vi "secondary_user.vi"() -> ()   [LabVIEW 2014]
uses:
  <vilib>/addons/Modulation/Digital/General/MT Generate Bits (Galois, PN Order).vi
  <vilib>/Analysis/7linalg.llb/Complex Eigenvalues and Vectors.vi
  <vilib>/Analysis/2dsp.llb/Complex FFT.vi
  <vilib>/addons/Modulation/Analog/support/mod_Set Error Source.vi
  <vilib>/addons/Modulation/Digital/Support/Common/Validators/mod_Generate Bits Validate.vi
  var_stop.vi
  <vilib>/addons/Modulation/Digital/Support/Common/Validators/mod_Generate Filter Coefficients Validate.vi
  <vilib>/addons/Modulation/Digital/General/subVIs/mod_Generate Filter Coefficients.vi
  <vilib>/measure/maspectr.llb/FFT Power Spectrum and PSD for 1 Chan (CDB).vi
  <vilib>/addons/Modulation/Digital/General/MT Apply Matched Filter (Generic).vi
  <vilib>/addons/Modulation/Digital/General/MT Align to Ideal Symbols (Generic).vi
  <vilib>/Analysis/7linalg.llb/Create Special Real Matrix.vi
  <vilib>/Analysis/Matrix/Numeric/Multiply/Multiply - RM,R.vi
  <vilib>/Analysis/Matrix/Numeric/Conversions/Matrix To Array - RM.vi
  <instrlib>/niUSRP/niUSRP Fetch Rx Data (CDB Cluster).vi
  <vilib>/Analysis/2dsp.llb/AutoCorrelation Matrix (CDB).vi
  <vilib>/Analysis/Matrix/Numeric/Multiply/Multiply - CM,C.vi
  <vilib>/Analysis/Matrix/Numeric/Conversions/Matrix To Array - CM.vi
  <vilib>/measure/madcrms.llb/Averaged DC-RMS for 1 Chan.vi
  <instrlib>/niUSRP/niUSRP Write Tx Data (CDB Cluster).vi
  <vilib>/addons/Modulation/Digital/General/subVIs/mod_Generate Bits PN Sequence.vi
  <vilib>/addons/Modulation/Digital/General/MT Apply Pulse Shaping Filter (Generic).vi
  <vilib>/addons/Modulation/niDMT.lvlib
  <vilib>/measure/NI_MAPro.lvlib
  <vilib>/Analysis/Matrix/NI_Matrix.lvlib
  <vilib>/Analysis/NI_AALPro.lvlib
  <vilib>/Analysis/NI_AAL_SigProc.lvlib
panel:
  in  "packet bits 2":i32[](array[numeric])
  in  "random bits 2":i8[](array[numeric])
  in  "Gray code? 2":bool
  in  "Modulation 2":enum16{"PSK", "QAM"}(ring)=enum."QAM"
  in  "filter length (symbols) 2":i32=8 caption="filter length (symbols)"
  in  "filter parameter 2":dbl=0.5 caption="filter parameter" format="%.2f"
  in  "pulse shaping filter (none) 2":T1(ring)=enum."Raised Cosine" caption="pulse shaping filter (none)"
  in  "M-PSK (4) 2":i32=4 caption="M-ARY"
  in  "samples per symbol (16) 2":i32=4 caption="samples per symbol (16)"
  out "RX coerced gain 2":dbl format="%#_6f"
  out "RX coerced carrier frequency 2":dbl=915000000.0 format="%#_6p"
  out "RX coerced IQ rate  2":dbl=4000000.0 format="%#_6p"
  in  "RX active antenna 2":string="RX2"
  in  "RX gain 2":dbl format="%#_6f"
  in  "RX device names 2":refnum<k15>="192.168.10.2"
  out "TX coerced gain 2":dbl format="%#_6f"
  out "TX coerced carrier frequency 2":dbl=915000000.0 format="%#_6p"
  out "coerced IQ rate 2":dbl=4000000.0 format="%#_6p"
  in  "TX device names 2":refnum<k15>="192.168.10.2"
  in  "TX gain 2":dbl format="%#_6f"
  in  "carrier frequency 2":dbl=915000000.0 format="%#_6p"
  in  "IQ rate 2":dbl=400000.0 format="%#_6p"
  in  "stop 2":bool
  in  "Send (deprecated) 2":bool
  in  "random bits length 2":i32=50000
  out "Numeric 4":i32
  in  "millisecond multiple 2":u32=1000
  in  "Keep sending 2":bool=TRUE caption="Keep sending"
  out "packet bits length 2":i32
  in  "Transmit power (db) 2":dbl
  out "x = y? 2":bool
  out "Numeric 3":i32
  in  "number of samples 2":i64=40000
  out "# elements in queue 2":i32
  out "packet len 2":u32
  out "RX Constellation Map 2":cdb[](graph)
  out "RX Constellation Map (uneq) 2":cdb[](graph)
  out "valid? 2":bool
  out "Spectrum monitor 2":cluster{"f0":dbl, "df":dbl, "magnitude":dbl[]}(graph)={"f0"=-0.49993781867926873, "df"=0.00012436264146250465, "magnitude"=[]}
  out "found? 2":bool
  out "Rx String 2":string
  out "error bits 2":i32
  out "received bits 2":i32
  out "ber 2":dbl
  out "error symbols 2":i32
  out "received symbols 2":dbl
  out "ser 2":dbl
  in  "Ratio of  redundant 2":i32=5
  out "Detection Noise":dbl
  out "Primary User's average signal":dbl
  out "Delta of gain":dbl format="%#_6f"
  in  "Detection Mode":bool=TRUE
  out "Noise Average":dbl
  out "Signal Average":dbl
  in  "Average size":i32=10
  in  "Noise Threshold":dbl=-105.0 format="%#_6f"
  in  "matrix type(Dont Change), need to be indentity":i32
  in  "order of AC matrix":i32=8
  out "df":dbl
  out "f0":dbl
  out "my average power":dbl
  out "Average Noise floor in dBm per Hz":dbl
  out "Eigenvalues":cdb[](array[numeric]) format="%.2f"
  out "Min Eigenvalue method":bool
  out "Minimum eigenvalue method":dbl
  out "Energy of the Signal":dbl
  out "min eigen value":dbl
  out "max eigen value":dbl
  out "Waveform Graph 2":dbl[](graph)
  out "Waveform Graph":dbl[](graph)
  out "Power Spectrum / PSD":cluster{"f0":dbl, "df":dbl, "magnitude":dbl[]}(graph)
  out "data":waveform(cdb)
  out "Noise floor in dBm per Hz":dbl
  out "Energy of the Signal in dBm per Hz":dbl
  in  "Keep sending":bool=TRUE
  in  "millisecond multiple":u32=1000
  out "Numeric 2":i32
  out "Numeric":i32
  out "x = y?":bool
  in  "Ratio of  redundant":i32=5
  out "ser":dbl
  out "received symbols":dbl
  out "error symbols":i32
  in  "random bits length":i32=50000
  in  "packet bits":i32[](array[numeric])
  out "RX Constellation Map (uneq)":cdb[](graph)
  in  "Transmit power (db)":dbl
  out "ber":dbl
  out "received bits":i32
  out "error bits":i32
  in  "random bits":i8[](array[numeric])
  out "found?":bool
  out "# elements in queue":i32
  out "Spectrum monitor":cluster{"f0":dbl, "df":dbl, "magnitude":dbl[]}(graph)={"f0"=-0.49993781867926873, "df"=0.00012436264146250465, "magnitude"=[]}
  out "RX Constellation Map":cdb[](graph)
  out "valid?":bool
  in  "Gray code?":bool
  in  "Modulation":enum16{"PSK", "QAM"}(ring)=enum."QAM"
  out "Rx String":string
  out "packet len":u32
  in  "Send (deprecated)":bool
  in  "filter length (symbols)":i32=8
  in  "filter parameter":dbl=0.5 format="%.2f"
  in  "pulse shaping filter (none)":T1(ring)=enum."Raised Cosine"
  in  "M-PSK (4)":i32=4 caption="M-ARY"
  in  "samples per symbol (16)":i32=4
  out "packet bits length":i32
  in  "number of samples":i64=40000
  out "RX coerced gain":dbl format="%#_6f"
  out "RX coerced carrier frequency":dbl=915000000.0 format="%#_6p"
  out "RX coerced IQ rate":dbl=4000000.0 format="%#_6p"
  in  "RX active antenna":string="RX2"
  in  "RX gain":dbl format="%#_6f"
  in  "RX device names":refnum<k15>="192.168.10.3"
  out "TX coerced gain":dbl format="%#_6f"
  out "TX coerced carrier frequency":dbl=915000000.0 format="%#_6p"
  out "coerced IQ rate":dbl=4000000.0 format="%#_6p"
  in  "TX device names":refnum<k15>="192.168.10.3"
  in  "TX gain":dbl format="%#_6f"
  in  "carrier frequency":dbl=915000000.0 format="%#_6p"
  in  "IQ rate":dbl=800000.0 format="%#_6p"
  in  "stop":bool
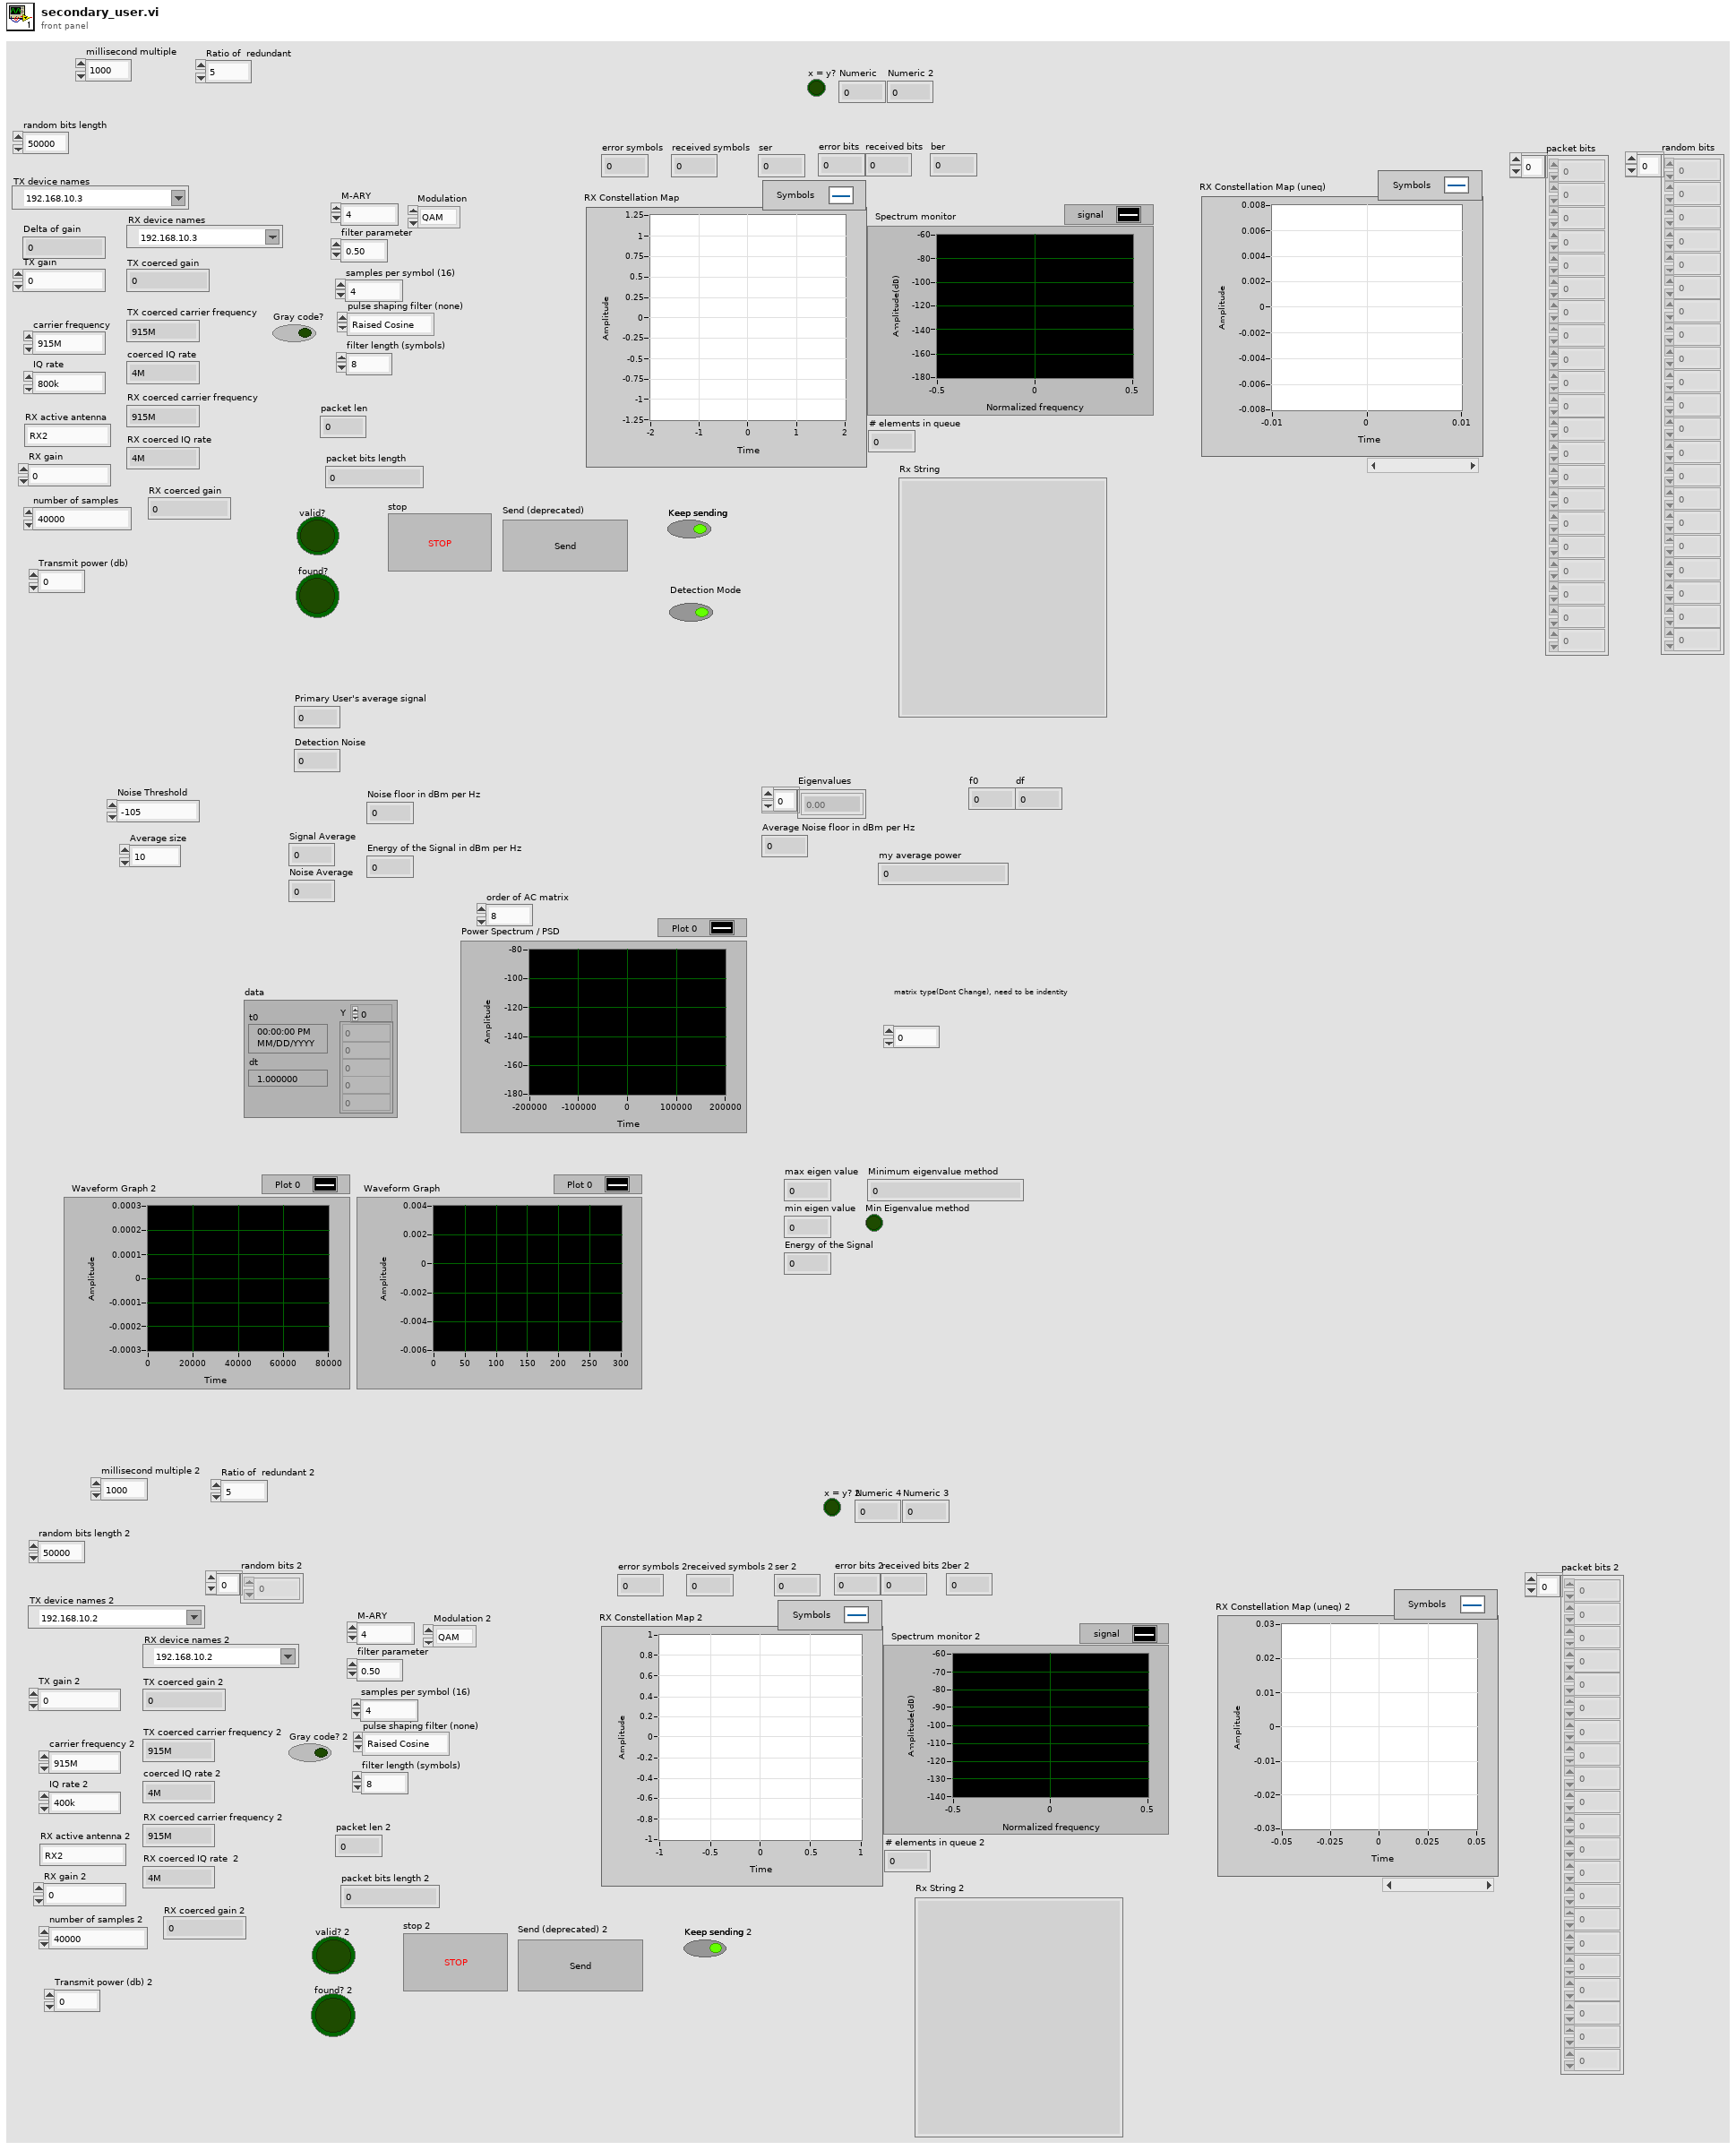
[diagram p1: front panel]
types:
  T1 = enum16{"none", "Raised Cosine", "Root Raised Cos", "Gaussian"}
  T2 = enum16{"FSK", "PSK", "QAM", "MSK", "PAM", "ASK", "CPM"}
  T3 = cluster{"samples per symbol (16)":i32, "symbol map":cdb[], "index map":u32[]}
  T4 = cluster{"samples per symbol (16)":i32, "symbol map":cdb[], i32[]}
  T5 = cluster{"samples per symbol (16) 2":i32, "symbol map":cdb[], "index map":u32[]}
  T6 = cluster{"samples per symbol (16) 2":i32, "symbol map":cdb[], i32[]}
  T7 = typedef "niAMT.lvlib/Complex Data Waveform.ctl" = cluster{"t0":dbl, "dt":dbl, "Y":cdb[]}
  T8 = typedef "NI_Matrix.lvlib/RealMatrix.ctl" = dbl[][]
  T9 = typedef "NI_Matrix.lvlib/ComplexMatrix.ctl" = cdb[][]
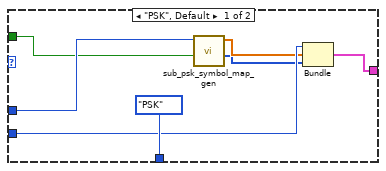
[diagram p2: hidden frame]
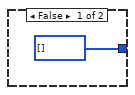
[diagram p5: hidden frame]
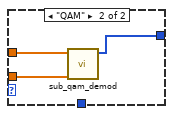
[diagram p6: hidden frame]
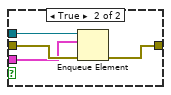
[diagram p10: hidden frame]
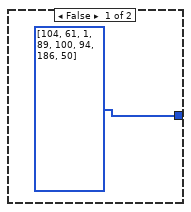
[diagram p13: hidden frame]
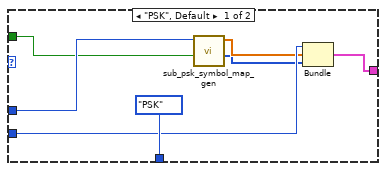
[diagram p18: hidden frame]
diagram:
  # "pre 64"
  # "Modulation"
  # "Filter"
  # "System Control"
  # "pre 64"
  # "Modulation"
  # "Filter"
  # "System Control"
  n1 = call <instrlib>:"niUSRP Open Rx Session.vi"("device names"="RX device names", "reset"=TRUE) -> ("session handle out"=w98:refnum<k15>, "error out"=w97:errorcluster)  [unwired: 12 in]
  n2 = call <instrlib>:"niUSRP Open Tx Session.vi"("device names"="TX device names", "reset"=TRUE) -> ("session handle out"=w110:refnum<k15>, "error out"=w109:errorcluster)  [unwired: 12 in]
  n3 = local read "Delta of gain"() -> (→"Delta of gain":dbl)
  n4 = call <instrlib>:"niUSRP Configure Signal.vi"("session handle"=w98, "IQ rate"="IQ rate", "carrier frequency"="carrier frequency", "gain"="RX gain", "error in (no error)"=w97, "active antenna"="RX active antenna") -> ("session handle out"=w89:refnum<k15>, "coerced IQ rate"=→"RX coerced IQ rate":dbl, "coerced carrier frequency"=→"RX coerced carrier frequency":dbl, "coerced gain"=→"RX coerced gain":dbl, "error out"=w73:errorcluster)  [unwired: 5 in]
  n5 = call <instrlib>:"niUSRP Open Rx Session.vi"("device names"="RX device names 2", "reset"=TRUE) -> ("session handle out"=w42:refnum<k15>, "error out"=w41:errorcluster)  [unwired: 12 in]
  n6 = call <instrlib>:"niUSRP Configure Signal.vi"("session handle"=w110, "IQ rate"="IQ rate", "carrier frequency"="carrier frequency", "gain"="TX gain", "error in (no error)"=w109, "active antenna"="TX1") -> ("session handle out"=w102:refnum<k15>, "coerced IQ rate"=w100:dbl, "coerced carrier frequency"=→"TX coerced carrier frequency":dbl, "coerced gain"=→"TX coerced gain":dbl, "error out"=w74:errorcluster)  [unwired: 5 in]
  "coerced IQ rate" <- w100
  n7 = case shown="\"QAM\"" "Modulation" {
    tunnel: [T2."PSK" ("modulation type") T2."QAM" ("modulation type")] -> w68
    tunnel: "M-PSK (4)" -> [w117 w123]
    tunnel: "Gray code?" -> [w116 w124]
    tunnel: "samples per symbol (16)" -> [w115 w122]
    tunnel: [w112 w119] -> w62
    frame "PSK", Default {
      n8 = call "sub_psk_symbol_map_gen.vi"("Gray code?"=w116, "M-PSK"=w117) -> ("index map"=w113:u32[], "symbol map"=w114:cdb[])  [unwired: 8 in]
      n9 = Bundle("samples per symbol (16)"=w115, "symbol map"=w114, "index map"=w113) -> (w112:T3)  [unwired: 1 in]
    }
    frame "QAM" {
      n10 = call "sub_qam_symbol_map_gen.vi"("Gray code?"=w124, "M-QAM"=w123) -> ("symbol map"=w121:cdb[])  [unwired: 9 in]
      n11 = Bundle("samples per symbol (16)"=w122, "symbol map"=w121, i32[] []) -> (w119:T4)  [unwired: 1 in]
    }
  }
  n12 = call <instrlib>:"niUSRP Open Tx Session.vi"("device names"="TX device names 2", "reset"=TRUE) -> ("session handle out"=w55:refnum<k15>, "error out"=w54:errorcluster)  [unwired: 12 in]
  n13 = call <vilib>:"MT Generate Filter Coefficients.vi"("pulse shaping filter (none)"="pulse shaping filter (none)", "modulation type"=w68, "pulse shaping samples per symbol (16)"="samples per symbol (16)", "matched samples per symbol (16)"="samples per symbol (16)", "filter parameter"="filter parameter", "filter length (symbols)"="filter length (symbols)") -> ("pulse shaping filter coefficients"=w79:dbl[], "matched filter coefficients"=w77:dbl[])  [unwired: 7 in, 1 out]
  n14 = call <instrlib>:"niUSRP Configure Signal.vi"("session handle"=w42, "IQ rate"="IQ rate 2", "carrier frequency"="carrier frequency 2", "gain"="RX gain 2", "error in (no error)"=w41, "active antenna"="RX active antenna 2") -> ("session handle out"=w33:refnum<k15>, "coerced IQ rate"=→"RX coerced IQ rate  2":dbl, "coerced carrier frequency"=→"RX coerced carrier frequency 2":dbl, "coerced gain"=→"RX coerced gain 2":dbl, "error out"=w17:errorcluster)  [unwired: 5 in]
  n15 = Unbundle(w62) -> ("symbol map"=w64:cdb[])  [unwired: 2 out]
  n16 = global write "var_stop.vi" "system stop"(FALSE) -> ()
  n17 = call "sub_bits_to_symbols.vi"("symbol map"=w64, "bits"=i16[] [1, 0, 1, 0, 1, 1, 0, 0, 1, 1, 0, 1, 1, 1, 0, 1, 1, 0, 1, 0, 0, 1, 0, 0, 1, 1, 1, 0, 0, 0, 1, 0, 1, 1, 1, 1, 0, 0, 1, 0, 1, 0, 0, 0, 1, 1, 0, 0, 0, 0, 1, 0, 0, 0, 0, 0, 1, 1, 1, 1, 1, 1, 0, 0] ("preamble(64) 2")) -> ("symbols"=w63:cdb[])  [unwired: 9 in]
  n18 = call <instrlib>:"niUSRP Configure Signal.vi"("session handle"=w55, "IQ rate"="IQ rate 2", "carrier frequency"="carrier frequency 2", "gain"="TX gain 2", "error in (no error)"=w54, "active antenna"="TX1") -> ("session handle out"=w46:refnum<k15>, "coerced IQ rate"=w44:dbl, "coerced carrier frequency"=→"TX coerced carrier frequency 2":dbl, "coerced gain"=→"TX coerced gain 2":dbl, "error out"=w18:errorcluster)  [unwired: 5 in]
  "coerced IQ rate 2" <- w44
  n19 = local write "packet bits"("packet bits") -> ()
  n20 = Divide(x="IQ rate", y="samples per symbol (16)") -> (x/y=w78:dbl)
  n21 = Merge Errors(w74, w73) -> (w72:errorcluster)
  n22 = local write "random bits"("random bits") -> ()
  n23 = case shown="\"QAM\"" "Modulation 2" {
    tunnel: [T2."PSK" ("modulation type") T2."QAM" ("modulation type")] -> w12
    tunnel: "M-PSK (4) 2" -> [w131 w137]
    tunnel: "Gray code? 2" -> [w130 w138]
    tunnel: "samples per symbol (16) 2" -> [w129 w136]
    tunnel: [w126 w133] -> w6
    frame "PSK", Default {
      n24 = call "sub_psk_symbol_map_gen.vi"("Gray code?"=w130, "M-PSK"=w131) -> ("index map"=w127:u32[], "symbol map"=w128:cdb[])  [unwired: 8 in]
      n25 = Bundle("samples per symbol (16) 2"=w129, "symbol map"=w128, "index map"=w127) -> (w126:T5)  [unwired: 1 in]
    }
    frame "QAM" {
      n26 = call "sub_qam_symbol_map_gen.vi"("Gray code?"=w138, "M-QAM"=w137) -> ("symbol map"=w135:cdb[])  [unwired: 9 in]
      n27 = Bundle("samples per symbol (16) 2"=w136, "symbol map"=w135, i32[] []) -> (w133:T6)  [unwired: 1 in]
    }
  }
  n28 = Reciprocal(x=w100) -> (1/x=w99:dbl)
  n29 = Obtain Queue(element data type=i8[] [] ("output bit stream")) -> (queue out=w84:refnum<queue>)  [unwired: 4 in, 2 out]
  n30 = Obtain Queue(element data type=i16[] []) -> (queue out=w111:refnum<queue>)  [unwired: 4 in, 2 out]
  n31 = Logarithm Base 2(1:"M-PSK (4)") -> (0:w59:dbl)
  n32 = Obtain Queue(element data type=cluster{"t0":dbl, "dt":dbl, "Y":cdb[]} {"t0"=0.0, "dt"=0.0, "Y"=[]} ("data")) -> (queue out=w88:refnum<queue>)  [unwired: 4 in, 2 out]
  n33 = Obtain Queue(element data type=cluster{"t0":dbl, "dt":dbl, "Y":cdb[]} {"t0"=0.0, "dt"=0.0, "Y"=[]} ("data")) -> (queue out=w85:refnum<queue>)  [unwired: 4 in, 2 out]
  n34 = Obtain Queue(element data type=cluster{"t0":dbl, "dt":dbl, "Y":cdb[]} {"t0"=0.0, "dt"=1.0, "Y"=[]} ("data")) -> (queue out=w103:refnum<queue>)  [unwired: 4 in, 2 out]
  n35 = call <vilib>:"MT Generate Filter Coefficients.vi"("pulse shaping filter (none)"="pulse shaping filter (none) 2", "modulation type"=w12, "pulse shaping samples per symbol (16)"="samples per symbol (16) 2", "matched samples per symbol (16)"="samples per symbol (16) 2", "filter parameter"="filter parameter 2", "filter length (symbols)"="filter length (symbols) 2") -> ("pulse shaping filter coefficients"=w23:dbl[], "matched filter coefficients"=w21:dbl[])  [unwired: 7 in, 1 out]
  n36 = case shown="No Error" w72 {
    tunnel: w111 -> [w190 _]
    tunnel: w103 -> [w185 _]
    tunnel: w102 -> [w186 _]
    tunnel: w99 -> [w144 _]
    tunnel: w89 -> [w175 _]
    tunnel: w88 -> [w169 _]
    tunnel: w85 -> [w165 _]
    tunnel: w84 -> [w163 _]
    tunnel: w62 -> [w157 _]
    tunnel: w79 -> [w160 _]
    tunnel: w78 -> [w159 _]
    tunnel: w77 -> [w158 _]
    tunnel: w63 -> [w151 _]
    tunnel: w59 -> [w149 _]
    frame No Error {
      w140 = 0
      w141 = 0.0
      w147 = 0
      w148 = 0
      # "USRP interface"
      n37 = call <instrlib>:"niUSRP Initiate.vi"("session handle"=w175, "error in (no error)"=errorcluster {"status"=FALSE, "code"=0, "source"=""}) -> ("session handle out"=w174:refnum<k15>, "error out"=w173:errorcluster)  [unwired: 12 in]
      n38 = while {
        tunnel: w163 -> [w212]
        shift-right: [w205] -> _
        shift-left: errorcluster {"status"=FALSE, "code"=0, "source"=""} ("error out") -> [w211]
        shift-right: [w200] -> _
        shift-left: w148 -> [w203]
        shift-right: [w201] -> _
        shift-left: w148 -> [w202]
        tunnel: w149 -> [w197]
        shift-right: [w194] -> _
        shift-left: w148 -> [w196]
        shift-right: [w193] -> _
        shift-left: w148 -> [w195]
        stop <- w210 stop-if-true
        n39 = Get Queue Status(queue=w212, error in (no error)=w211) -> (queue out=w207:refnum<queue>, error out=w206:errorcluster, # elements in queue=w209:i32)  [unwired: 1 in, 5 out]
        n40 = local read "packet bits length"() -> (w198:i32)
        n41 = local read "random bits"() -> (w204:i8[])
        n42 = Not Equal To 0?(x=w209) -> (x != 0?=w208:bool)
        n43 = case shown="True" w208 {
          tunnel: w207 -> [_ w254]
          tunnel: w206 -> [w217 w253]
          tunnel: [w217 w248] -> w205
          tunnel: w204 -> [_ w245]
          tunnel: w203 -> [w216 w241]
          tunnel: [w216 w240] -> w200
          tunnel: [w215 w238] -> w201
          tunnel: w202 -> [w215 w239]
          tunnel: w198 -> [_ w230]
          tunnel: w197 -> [_ w226]
          tunnel: w196 -> [w214 w222]
          tunnel: [w214 w221] -> w194
          tunnel: w195 -> [w213 w220]
          tunnel: [w213 w218] -> w193
          frame False {
          }
          frame True {
            w234 = 0
            w251 = 8 ("y")
            n44 = Dequeue Element(queue=w254, error in (no error)=w253) -> (element=w231:i8[], error out=w248:errorcluster)  [unwired: 1 in, 2 out]
            n45 = Array Size(array=w231) -> (size(s)=w225:i32)
            n46 = Subtract(x=w230, y=w225) -> (x-y=w229:i32)
            n47 = Array Subset(array=w245, index=0, length=w225) -> (w232:i8[])
            n48 = Quotient & Remainder(x=w229, y=w226) -> (x-y*floor(x/y)=w235:dbl)  [unwired: 1 out]
            n49 = Not Equal?(x=w232, y=w231) -> (x != y?=w244:bool[])
            n50 = Initialize Array(0, w235) -> (w233:i32[])
            n51 = Boolean To (0,1)(Boolean=w244) -> (0, 1=w243:i16[])
            n52 = Add Array Elements(numeric array=w243) -> (sum=w242:i16)
            n53 = Quotient & Remainder(x=w225, y=w226) -> (floor(x/y)=w219:dbl)  [unwired: 1 out]
            n54 = Insert Into Array(array=w233, index=w234, new element=w232) -> (w228:i32[])
            n55 = Insert Into Array(array=w233, index=w234, new element=w231) -> (w227:i32[])
            n56 = Quotient & Remainder(x=w225, y=w251) -> (floor(x/y)=w250:i32)  [unwired: 1 out]
            n57 = Add(x=w241, y=w242) -> (x+y=w240:i32)
            n58 = Add(x=w239, y=w225) -> (x+y=w238:i32)
            n59 = Not Equal To 0?(x=w231) -> (x != 0?=w252:bool[])
            n60 = Reshape Array(w228, w219, w226) -> (w224:i32[][])
            n61 = Reshape Array(w227, w219, w226) -> (w223:i32[][])
            n62 = Add(x=w219, y=w220) -> (x+y=w218:dbl)
            n63 = Reshape Array(w252, w250, w251) -> (w249:bool[][])
            n64 = for {
              tunnel: w224 -> [w262] mode=indexing
              tunnel: w223 -> [w263] mode=indexing
              shift-right: [w258] -> w221
              shift-left: w222 -> [w257]
              n65 = Not Equal?(x=w262, y=w263) -> (x != y?=w261:bool[])
              n66 = Boolean To (0,1)(Boolean=w261) -> (0, 1=w260:i16[])
              n67 = Add Array Elements(numeric array=w260) -> (sum=w259:i16)
              n68 = Not Equal To 0?(x=w259) -> (x != 0?=w256:bool)
              n69 = Boolean To (0,1)(Boolean=w256) -> (0, 1=w255:i16)
              n70 = Add(x=w255, y=w257) -> (x+y=w258:i32)
            }
            n71 = for {
              tunnel: w249 -> [w266] mode=indexing
              tunnel: [w265] -> w247 mode=indexing
              n72 = Boolean Array To Number(Boolean array=w266) -> (number=w264:u32)
              n73 = To Unsigned Byte Integer(number=w264) -> (unsigned 8bit integer=w265:u8)
            }
            n74 = Byte Array To String(unsigned byte array=w247) -> (string=→"Rx String":string)
          }
        }
        "error bits" <- w200
        "received bits" <- w201
        "error symbols" <- w194
        "received symbols" <- w193
        n75 = Divide(x=w194, y=w193) -> (x/y=→"ser":dbl)
        n76 = Divide(x=w200, y=w201) -> (x/y=→"ber":dbl)
        n77 = global read "var_stop.vi" "system stop"() -> (w210:bool)
      }
      n78 = while {
        tunnel: w169 -> [w359]
        shift-right: [w352] -> _
        shift-left: errorcluster {"status"=FALSE, "code"=0, "source"=""} ("error out") -> [w358]
        shift-right: [w338] -> _
        shift-left: cluster{"t0":dbl, "dt":dbl, "Y":cdb[]} {"t0"=0.0, "dt"=0.0, "Y"=[]} ("data") -> [w353]
        tunnel: w165 -> [w351]
        shift-right: [w350] -> _
        shift-left: errorcluster {"status"=FALSE, "code"=0, "source"=""} ("error out") -> [w349]
        stop <- w348 stop-if-true
        # "Energy\ndetector"
        n79 = Get Queue Status(queue=w359, error in (no error)=w358) -> (queue out=w354:refnum<queue>, error out=w355:errorcluster, # elements in queue=w357:i32)  [unwired: 1 in, 5 out]
        n80 = Not Equal To 0?(x=w357) -> (x != 0?=w356:bool)
        n81 = case shown="True" w356 {
          tunnel: w355 -> [w381 w392]
          tunnel: w354 -> [_ w391]
          tunnel: w353 -> [w380 w386]
          tunnel: [w381 w383] -> w352
          tunnel: [w380 w382] -> w345
          frame False {
          }
          frame True {
            n82 = Unbundle(w386) -> ("Y"=w389:cdb[])  [unwired: 2 out]
            n83 = Dequeue Element(queue=w391, error in (no error)=w392) -> (element=w390:cluster{"t0":dbl, "dt":dbl, "Y":cdb[]}, error out=w383:errorcluster)  [unwired: 1 in, 2 out]
            n84 = Unbundle(w390) -> ("t0"=w385:dbl, "dt"=w384:dbl, "Y"=w388:cdb[])
            n85 = Build Array (concatenate)(w389, w388) -> (w387:cdb[])
            n86 = Bundle(cluster=w386, "t0"=w385, "dt"=w384, "Y"=w387) -> (w382:cluster{"t0":dbl, "dt":dbl, "Y":cdb[]})
          }
        }
        n87 = call "rx_ed.vi"("Wavefrom"=w345) -> ("first pulse"=w335:i32, "length"=w346:i32[], "start index"=w347:i32[])  [unwired: 8 in]
        n88 = for {
          tunnel: w351 -> [w367]
          tunnel: w345 -> [w364]
          shift-right: [w366] -> w350
          shift-left: w349 -> [w365]
          tunnel: w347 -> [w363] mode=indexing
          tunnel: w346 -> [w362] mode=indexing
          tunnel: [w363] -> w341
          tunnel: [w362] -> w340
          n89 = Greater Or Equal?(x=w362, y=128) -> (x >= y?=w360:bool)
          n90 = case shown="True" w360 {
            tunnel: w367 -> [_ w379]
            tunnel: [w368 w378] -> w366
            tunnel: w365 -> [w368 w377]
            tunnel: w364 -> [_ w376]
            tunnel: w363 -> [_ w370]
            tunnel: w362 -> [_ w369]
            frame False {
            }
            frame True {
              n91 = Unbundle(w376) -> ("t0"=w374:dbl, "dt"=w375:dbl, "Y"=w372:cdb[])
              n92 = Array Subset(array=w372, index=w370, length=w369) -> (w371:cdb[])
              n93 = Bundle("t0"=w374, "dt"=w375, w371) -> (w373:cluster{"t0":dbl, "dt":dbl, cdb[]})  [unwired: 1 in]
              n94 = Enqueue Element(queue=w379, element=w373, error in (no error)=w377) -> (error out=w378:errorcluster)  [unwired: 1 in, 2 out]
            }
          }
        }
        n95 = Add(x=w341, y=w340) -> (x+y=w337:i32)
        n96 = Max & Min(x=w337, y=w335) -> (max(x,y)=w336:i32)  [unwired: 1 out]
        n97 = Unbundle(w345) -> ("t0"=w344:dbl, "dt"=w343:dbl, "Y"=w342:cdb[])
        n98 = global read "var_stop.vi" "system stop"() -> (w348:bool)
        n99 = Array Subset(array=w342, index=w336) -> (w339:cdb[])  [unwired: 1 in]
        n100 = Bundle(cluster=w345, "t0"=w344, "dt"=w343, "Y"=w339) -> (w338:cluster{"t0":dbl, "dt":dbl, "Y":cdb[]})
      }
      n101 = while {
        tunnel: w165 -> [w280]
        shift-right: [w274] -> _
        shift-left: errorcluster {"status"=FALSE, "code"=0, "source"=""} ("error out") -> [w279]
        tunnel: w163 -> [w273]
        shift-right: [w272] -> _
        shift-left: errorcluster {"status"=FALSE, "code"=0, "source"=""} ("error out") -> [w271]
        tunnel: w158 -> [w269]
        tunnel: w157 -> [w268]
        tunnel: w151 -> [w267]
        stop <- w270 stop-if-true
        # "Signal \nDemodulator"
        n102 = Get Queue Status(queue=w280, error in (no error)=w279) -> (queue out=w276:refnum<queue>, error out=w275:errorcluster, # elements in queue=w278:i32)  [unwired: 1 in, 5 out]
        n103 = Not Equal To 0?(x=w278) -> (x != 0?=w277:bool)
        n104 = case shown="True" w277 {
          tunnel: w276 -> [_ w313]
          tunnel: w275 -> [w282 w314]
          tunnel: [w282 w312] -> w274
          tunnel: w273 -> [_ w305]
          tunnel: [w281 w304] -> w272
          tunnel: w271 -> [w281 w303]
          tunnel: w269 -> [_ w292]
          tunnel: w268 -> [_ w296]
          tunnel: w267 -> [_ w288]
          frame False {
          }
          frame True {
            # "cross+eq"
            n105 = Unbundle(w296) -> ("samples per symbol (16)"=w295:i32, "symbol map"=w294:cdb[], "index map"=w293:u32[])
            n106 = Dequeue Element(queue=w313, error in (no error)=w314) -> (element=w287:cluster{"t0":dbl, "dt":dbl, "Y":cdb[]}, error out=w312:errorcluster)  [unwired: 1 in, 2 out]
            n107 = Unbundle(w287) -> ("Y"=w286:cdb[])  [unwired: 2 out]
            n108 = Bundle By Name("Y"=w286) -> (w291:waveform(cdb))  [unwired: 1 in]
            n109 = call-poly <vilib>:"FFT Power Spectrum and PSD.vi"("dB On (F)"=TRUE, "time signal"=w291) -> ("Power Spectrum / PSD"=→"Spectrum monitor":cluster{"f0":dbl, "df":dbl, "magnitude":dbl[]})  [unwired: 6 in, 3 out]
            n110 = call-poly <vilib>:"MT Matched Filter.vi"("input complex waveform"=w287, "matched filter coefficients"=w292, "samples per symbol (16)"=w295, "reset? (T)"=FALSE) -> ("output complex waveform"=w311:T7, "error out"=w310:errorcluster)  [unwired: 10 in]
            n111 = call-poly <vilib>:"MT Align To Ideal Symbols.vi"("input complex waveform"=w311, "matched filter coefficients"=w292, "samples per symbol (16)"=w295, "error in (no error)"=w310, "reset? (T)"=FALSE) -> ("output complex waveform"=w308:T7, "error out"=w309:errorcluster)  [unwired: 8 in, 1 out]
            n112 = call <vilib>:"MT Decimate Oversampled Waveform.vi"("input complex waveform"=w308, "decimation factor"=w295, "error in (no error)"=w309, "reset? (T)"=FALSE) -> ("output complex waveform"=w307:T7)  [unwired: 10 in, 1 out]
            n113 = Unbundle(w307) -> ("Y"=w285:cdb[])  [unwired: 2 out]
            n114 = call "rx_ceEq.vi"("preamble"=w288, "symbols"=w285) -> ("valid?"=w301:bool, "eq symbols"=w302:cdb[])
            "valid?" <- w301
            n115 = case shown="True" w301 {
              tunnel: [i8[] [] ("output bit stream") w319] -> w284
              tunnel: w294 -> [_ w320]
              tunnel: w302 -> [_ w317]
              tunnel: w293 -> [_ w318]
              tunnel: w285 -> [_ w316]
              frame False {
              }
              frame True {
                n116 = local read "Modulation"() -> (w321:enum16{"PSK", "QAM"})
                n117 = case shown="\"PSK\", Default" w321 {
                  tunnel: w317 -> [w325 w328]
                  tunnel: w320 -> [w324 w327]
                  tunnel: [w322 w326] -> w319
                  tunnel: w318 -> [w323 _]
                  frame "PSK", Default {
                    n118 = call "sub_psk_demod.vi"("index map"=w323, "symbol map"=w324, "symbol"=w325) -> ("bitstream"=w322:i16[])  [unwired: 8 in]
                  }
                  frame "QAM" {
                    n119 = call "sub_qam_demod.vi"("symbol map"=w327, "symbol"=w328) -> ("bitstream"=w326:i16[])  [unwired: 9 in]
                  }
                }
                "RX Constellation Map" <- w317
                "RX Constellation Map (uneq)" <- w316
              }
            }
            n120 = call "rx_pduExtract.vi"("output bit stream"=w284) -> ("found?"=w306:bool, "packet len"=w300:u32, "ppdu"=w283:i8[])  [unwired: 2 in]
            "found?" <- w306
            n121 = case shown="True" w306 {
              tunnel: w283 -> [_ w332]
              tunnel: w305 -> [_ w334]
              tunnel: [w329 w333] -> w304
              tunnel: w303 -> [w329 w330]
              tunnel: w300 -> [_ w331]
              frame False {
              }
              frame True {
                n122 = Enqueue Element(queue=w334, element=w332, error in (no error)=w330) -> (error out=w333:errorcluster)  [unwired: 1 in, 2 out]
                "packet len" <- w331
              }
            }
          }
        }
        n123 = global read "var_stop.vi" "system stop"() -> (w270:bool)
      }
      n124 = Initialize Array(cdb 0.0+0.0i, 25000 ("dimension size")) -> (w180:cdb[])
      n125 = Initialize Array(w141, w140) -> (w142:dbl[])
      n126 = while {
        tunnel: w190 -> [w690]
        shift-right: [w688] -> _
        shift-left: errorcluster {"status"=FALSE, "code"=0, "source"=""} ("error out") -> [w689]
        shift-right: [w686] -> _
        shift-left: -1111 -> [w687]
        shift-right: [w684] -> _
        shift-left: w147 -> [w685]
        tunnel: "Ratio of  redundant" -> [w683]
        stop <- "stop" stop-if-true
        n127 = local write "Detection Mode"("Detection Mode") -> ()
        n128 = Wait Until Next ms Multiple(millisecond multiple="millisecond multiple") -> ()  [unwired: 1 out]
        n129 = global write "var_stop.vi" "system stop"("stop") -> ()
        n130 = Not(x="Detection Mode") -> (.not. x?=w679:bool)
        n131 = And(x="Keep sending", y=w679) -> (x .and. y?=w681:bool)
        n132 = case shown="True" w681 {
          tunnel: w690 -> [_ w715]
          tunnel: w689 -> [w694 w714]
          tunnel: [w694 w713] -> w688
          tunnel: w687 -> [w693 w710]
          tunnel: [w693 w709] -> w686
          tunnel: w685 -> [w692 w695]
          tunnel: [w692 w700] -> w684
          tunnel: w683 -> [_ w701]
          frame False {
          }
          frame True {
            w707 = 8
            n133 = call-poly <vilib>:"MT Generate Bits (poly).vi"("total bits (128)"="random bits length", "seed in (0xD6BF7DF2)"=w710, "reset? (T)"=FALSE) -> ("output bit stream"=w697:i8[], "seed out"=w709:i32)  [unwired: 10 in, 1 out]
            n134 = Not Equal To 0?(x=w697) -> (x != 0?=w702:bool[])
            n135 = Array Size(array=w702) -> (size(s)=w706:i32)
            n136 = Divide(x=w706, y=w707) -> (x/y=w705:dbl)
            n137 = Reshape Array(w702, w705, w707) -> (w704:bool[][])
            n138 = for {
              tunnel: w704 -> [w720] mode=indexing
              tunnel: [w718] -> w703 mode=indexing
              n139 = Boolean Array To Number(Boolean array=w720) -> (number=w719:u32)
              n140 = To Unsigned Byte Integer(number=w719) -> (unsigned 8bit integer=w718:u8)
            }
            n141 = Increment(x=w695) -> (x+1=w700:i32)
            n142 = Array Size(array=w703) -> (size(s)=w712:i32)
            n143 = Quotient & Remainder(x=w695, y=w701) -> (x-y*floor(x/y)=w696:i32)  [unwired: 1 out]
            n144 = Not Equal To 0?(x=w712) -> (x != 0?=w716:bool)
            n145 = Equal?(x=w696, y=0) -> (x = y?=w698:bool)
            n146 = case shown="True" w716 {
              tunnel: w703 -> [_ w722]
              tunnel: w715 -> [_ w725]
              tunnel: w714 -> [w721 w724]
              tunnel: [w721 w723] -> w713
              frame False {
              }
              frame True {
                n147 = Enqueue Element(queue=w725, element=w722, error in (no error)=w724) -> (error out=w723:errorcluster)  [unwired: 1 in, 2 out]
              }
            }
            n148 = case shown="True" w698 {
              tunnel: w697 -> [_ w717]
              frame False {
              }
              frame True {
                n149 = local write "random bits"(w717) -> ()
              }
            }
            "Numeric" <- w695
          }
        }
      }
      n150 = while {
        tunnel: w174 -> [w513]
        shift-right: [w503] -> w170
        shift-left: w173 -> [w512]
        tunnel: w169 -> [w511]
        shift-right: [w505] -> _
        shift-left: errorcluster {"status"=FALSE, "code"=0, "source"=""} ("error out") -> [w510]
        tunnel: [w504] -> w171
        shift-right: [w447] -> _
        shift-left: errorcluster {"status"=FALSE, "code"=0, "source"=""} ("error out") -> [w448]
        shift-right: [w441] -> _
        shift-left: w141 -> [w442]
        shift-right: [w439] -> _
        shift-left: w140 -> [w440]
        tunnel: w144 -> [w435]
        tunnel: "Noise Threshold" -> [w422]
        shift-right: [w416] -> _
        shift-left: w142 -> [w420]
        shift-right: [w415] -> _
        shift-left: w142 -> [w419]
        shift-right: [w414] -> _
        shift-left: w141 -> [w418]
        shift-right: [w413] -> _
        shift-left: w141 -> [w417]
        shift-right: [w409] -> _
        shift-left: w141 -> [w411]
        shift-right: [w410] -> _
        shift-left: w141 -> [w397]
        shift-right: [w403] -> _
        shift-left: w140 -> [w405]
        shift-right: [w395] -> _
        shift-left: w141 -> [w396]
        i -> [w501]
        stop <- w502 stop-if-true
        # "USRP\nReceiver"
        n151 = local read "Detection Mode"() -> (w394:bool)
        n152 = Increment(x=w440) -> (x+1=w439:i32)
        n153 = Get Queue Status(queue=w511, error in (no error)=w510) -> (queue out=w507:refnum<queue>, error out=w506:errorcluster, # elements in queue=w509:i32)  [unwired: 1 in, 5 out]
        "# elements in queue" <- w509
        n154 = Less?(x=w509, y=5000) -> (x < y?=w499:bool)
        n155 = Greater Or Equal?(x=w501, y=25) -> (x >= y?=w498:bool)
        n156 = call-poly <vilib>:"Create Special Matrix.vi"("matrix type"="matrix type(Dont Change), need to be indentity", "matrix size"="order of AC matrix") -> ("Special Matrix"=w443:T8)  [unwired: 3 in, 1 out]
        n157 = And(x=w499, y=w498) -> (x .and. y?=w497:bool)
        n158 = call-poly <instrlib>:"niUSRP Fetch Rx Data (poly).vi"("session handle"=w513, "number of samples"="number of samples", "error in (no error)"=w512) -> ("session handle out"=w504:refnum<k15>, "data"=w462:cluster{"t0":dbl, "dt":dbl, "Y":cdb[]}, "error out"=w503:errorcluster)  [unwired: 9 in, 1 out]
        n159 = case shown="False" w497 {
          tunnel: w507 -> [_ w588]
          tunnel: w506 -> [w584 w587]
          tunnel: [w584 w586] -> w505
          tunnel: w462 -> [_ w585]
          frame False {
          }
          frame True {
            n160 = Enqueue Element(queue=w588, element=w585, error in (no error)=w587) -> (error out=w586:errorcluster)  [unwired: 1 in, 2 out]
          }
        }
        n161 = Unbundle(w462) -> ("dt"=w479:dbl, "Y"=w393:cdb[])  [unwired: 1 out]
        n162 = call-poly <vilib>:"AutoCorrelation Matrix.vi"("order"="order of AC matrix", "X"=w393) -> ("AutoCorrelation Matrix"=w444:T9)  [unwired: 8 in, 1 out]
        n163 = Absolute Value(x=w393) -> (abs(x)=w438:dbl[])
        n164 = Square(x=w438) -> (x^2=w481:dbl[])
        n165 = Add Array Elements(numeric array=w481) -> (sum=w473:dbl)
        "Energy of the Signal" <- w473
        n166 = Bundle By Name("Y"=w393, "dt"=w479) -> (w476:waveform(cdb))  [unwired: 1 in]
        "data" <- w476
        "Waveform Graph 2" <- w476
        n167 = Multiply(x=w473, y=w435) -> (x*y=w495:dbl)
        n168 = call-poly <vilib>:"Multiply.vi"("Complex Scalar c"=w435, "Complex Matrix A"=w444) -> ("A * c"=w487:T9)
        n169 = call-poly <vilib>:"Multiply.vi"("Real Scalar c"=2.05717e-20, "Real Matrix A"=w443) -> ("A * c"=w488:T8)
        n170 = Divide(x=w495, y="number of samples") -> (x/y=w463:dbl)
        n171 = call-poly <vilib>:"Matrix To Array.vi"("Complex Matrix"=w487) -> ("Complex 2D Array"=w489:cdb[][])
        n172 = call-poly <vilib>:"Matrix To Array.vi"("Real Matrix"=w488) -> ("Real 2D Array"=w490:dbl[][])
        n173 = Multiply(x=w463, y=1000.0) -> (x*y=w423:dbl)
        n174 = call-poly <vilib>:"FFT Power Spectrum and PSD.vi"("error in (no error)"=w448, "dB On (F)"=TRUE ("reset? (T)"), "time signal"=w476) -> ("error out"=w470:errorcluster, "Power Spectrum / PSD"=w449:cluster{"f0":dbl, "df":dbl, "magnitude":dbl[]})  [unwired: 5 in, 2 out]
        "Power Spectrum / PSD" <- w449
        n175 = Logarithm Base 10(1:w423) -> (0:w483:dbl)
        n176 = Logarithm Base 10(1:w423) -> (0:w425:dbl)
        n177 = Add(x=w489, y=w490) -> (x+y=w491:cdb[][])
        n178 = Multiply(x=w483, y=10.0) -> (x*y=→"Energy of the Signal in dBm per Hz":dbl)
        n179 = Multiply(x=w425, y=10.0) -> (x*y=w424:dbl)
        n180 = call-poly <vilib>:"Eigenvalues and Vectors.vi"("Input Matrix"=w491) -> ("Eigenvalues"=w492:cdb[])  [unwired: 2 in, 2 out]
        "Eigenvalues" <- w492
        n181 = Unbundle(w449) -> ("f0"=→"f0":dbl, "df"=→"df":dbl, "magnitude"=w456:dbl[])
        n182 = Absolute Value(x=w492) -> (abs(x)=w496:dbl[])
        n183 = Greater?(x=w424, y=w422) -> (0:w421:bool)
        n184 = case shown="True" w421 {
          tunnel: w420 -> [w544 w570]
          tunnel: w419 -> [w546 w566]
          tunnel: "Average size" -> [w545 w572]
          tunnel: w423 -> [w539 w563]
          tunnel: [w544 w567] -> w416
          tunnel: [w543 w566] -> w415
          tunnel: w418 -> [w542 w562]
          tunnel: w417 -> [w540 w565]
          tunnel: [w541 w565] -> w413
          tunnel: [w542 w564] -> w414
          tunnel: w405 -> [w537 w559]
          tunnel: w394 -> [_ w560]
          tunnel: [w537 w558] -> w403
          frame False {
            n185 = Add(x=w539, y=w540) -> (x+y=w538:dbl)
            n186 = Array Size(array=w546) -> (size(s)=w547:i32)
            n187 = Greater Or Equal?(x=w547, y=w545) -> (x >= y?=w548:bool)
            n188 = case shown="True" w548 {
              tunnel: w546 -> [w552 w557]
              tunnel: [w552 w556] -> w549
              tunnel: w538 -> [w551 w555]
              tunnel: [w551 w553] -> w541
              frame False {
              }
              frame True {
                n189 = Delete From Array(array=w557) -> (deleted portion=w554:dbl, array with subset deleted=w556:dbl[])  [unwired: 2 in]
                n190 = Subtract(x=w555, y=w554) -> (x-y=w553:dbl)
              }
            }
            n191 = Insert Into Array(array=w549, index=0, new element=w539) -> (w543:dbl[])
          }
          frame True {
            n192 = Array Size(array=w570) -> (size(s)=w573:i32)
            n193 = Add(x=w563, y=w562) -> (x+y=w561:dbl)
            n194 = Greater Or Equal?(x=w573, y=w572) -> (x >= y?=w571:bool)
            n195 = case shown="True" w571 {
              tunnel: w570 -> [w578 w583]
              tunnel: [w578 w582] -> w569
              tunnel: w561 -> [w577 w581]
              tunnel: [w577 w579] -> w564
              frame False {
              }
              frame True {
                n196 = Delete From Array(array=w583) -> (deleted portion=w580:dbl, array with subset deleted=w582:dbl[])  [unwired: 2 in]
                n197 = Subtract(x=w581, y=w580) -> (x-y=w579:dbl)
              }
            }
            n198 = case shown="False" w560 {
              tunnel: [w574 w576] -> w558
              tunnel: w559 -> [w575 w576]
              frame False {
                n199 = Increment(x=w575) -> (x+1=w574:i32)
              }
              frame True {
              }
            }
            n200 = Insert Into Array(array=w569, index=0, new element=w563) -> (w567:dbl[])
          }
        }
        n201 = Divide(x=w456, y=10.0) -> (x/y=w457:dbl[])
        n202 = Array Max & Min(array=w496) -> (max value=→"max eigen value":dbl, min value=w468:dbl)  [unwired: 2 out]
        "min eigen value" <- w468
        n203 = call-poly <vilib>:"Averaged DC-RMS.vi"("error in (no error)"=w470, "signal in"=w476) -> ("error out"=w447:errorcluster)  [unwired: 5 in, 4 out]
        n204 = Array Size(array=w456) -> (size(s)=w460:i32)
        n205 = Divide(x=w473, y=w468) -> (x/y=w437:dbl)
        "Minimum eigenvalue method" <- w437
        n206 = Power Of 10(x=w457) -> (10^x=w454:dbl[])
        n207 = Logarithm Base 10(1:w468) -> (0:w493:dbl)
        n208 = Greater?(x=w437, y=800000000000000.0) -> (0:→"Min Eigenvalue method":bool)
        n209 = Add Array Elements(numeric array=w454) -> (sum=w461:dbl)
        n210 = call-poly <vilib>:"FFT.vi"("FFT size"=256, "shift?"=FALSE, "X"=w393) -> ("FFT {X}"=→"Waveform Graph":cdb[])  [unwired: 7 in, 1 out]
        n211 = Divide(x=w461, y=w460) -> (x/y=w453:dbl)
        n212 = Multiply(x=w493, y=10.0) -> (x*y=→"Noise floor in dBm per Hz":dbl)
        n213 = Logarithm Base 10(1:w453) -> (0:w452:dbl)
        n214 = Array Size(array=w416) -> (size(s)=w429:i32)
        n215 = Multiply(x=w452, y=10.0) -> (x*y=→"my average power":dbl)
        n216 = Quotient & Remainder(x=w403, y="Average size") -> (x-y*floor(x/y)=w402:i32)  [unwired: 1 out]
        n217 = Divide(x=w414, y=w429) -> (x/y=w430:dbl)
        n218 = Equal To 0?(x=w402) -> (x = 0?=w400:bool)
        n219 = Not Equal To 0?(x=w397) -> (x != 0?=w408:bool)
        n220 = Logarithm Base 10(1:w430) -> (0:w433:dbl)
        n221 = And(x=w394, y=w408) -> (x .and. y?=w406:bool)
        n222 = global read "var_stop.vi" "system stop"() -> (w502:bool)
        n223 = Multiply(x=w433, y=10.0) -> (x*y=w398:dbl)
        "Signal Average" <- w398
        n224 = Add(x=w468, y=w442) -> (x+y=w441:dbl)
        n225 = Not Equal To 0?(x=w398) -> (x != 0?=w407:bool)
        n226 = Divide(x=w441, y=w439) -> (x/y=w467:dbl)
        n227 = And(x=w407, y=w406) -> (x .and. y?=w401:bool)
        n228 = Logarithm Base 10(1:w467) -> (0:w466:dbl)
        n229 = Array Size(array=w415) -> (size(s)=w428:i32)
        n230 = And(x=w400, y=w401) -> (x .and. y?=w399:bool)
        n231 = Multiply(x=w466, y=10.0) -> (x*y=→"Average Noise floor in dBm per Hz":dbl)
        n232 = case shown="True" w399 {
          tunnel: w398 -> [_ w524]
          tunnel: w397 -> [_ w523]
          tunnel: w396 -> [w514 w520]
          tunnel: [w514 w515] -> w395
          frame False {
          }
          frame True {
            n233 = Subtract(x=w524, y=w523) -> (x-y=w517:dbl)
            n234 = Greater Than 0?(x=w517) -> (x > 0?=w522:bool)
            n235 = Add(x=w517, y=10.0) -> (x+y=w519:dbl)
            n236 = case shown="True" w522 {
              tunnel: w517 -> [_ w531]
              tunnel: w520 -> [w529 w532]
              tunnel: [w529 w530] -> w516
              frame False {
              }
              frame True {
                n237 = Subtract(x=w532, y=w531) -> (x-y=w530:dbl)
              }
            }
            n238 = Less Than 0?(x=w519) -> (x < 0?=w518:bool)
            n239 = case shown="False" w518 {
              tunnel: w517 -> [_ w527]
              tunnel: w516 -> [w525 w528]
              tunnel: [w525 w526] -> w515
              frame False {
              }
              frame True {
                n240 = Subtract(x=w528, y=w527) -> (x-y=w526:dbl)
              }
            }
          }
        }
        n241 = Divide(x=w413, y=w428) -> (x/y=w427:dbl)
        n242 = Logarithm Base 10(1:w427) -> (0:w431:dbl)
        n243 = Multiply(x=w431, y=10.0) -> (x*y=w412:dbl)
        "Noise Average" <- w412
        n244 = case shown="True" w394 {
          tunnel: w398 -> [_ w536]
          tunnel: w412 -> [_ w535]
          tunnel: w411 -> [w534 _]
          tunnel: [w533 w535] -> w410
          tunnel: w397 -> [w533 _]
          tunnel: [w534 w536] -> w409
          frame False {
          }
          frame True {
          }
        }
        "Primary User's average signal" <- w409
        "Detection Noise" <- w410
        n245 = local write "Delta of gain"(w395) -> ()
      }
      n246 = Bundle(0.0, w144, w180) -> (w178:cluster{dbl, dbl, cdb[]})  [unwired: 1 in]
      n247 = while {
        shift-right: [w598] -> w189
        shift-left: errorcluster {"status"=FALSE, "code"=0, "source"=""} ("error out") -> [w596]
        tunnel: [w597] -> w188
        tunnel: w186 -> [w595]
        tunnel: w185 -> [w593]
        shift-right: [w591] -> _
        shift-left: errorcluster {"status"=FALSE, "code"=0, "source"=""} ("error out") -> [w592]
        tunnel: w178 -> [w590]
        stop <- w589 stop-if-true
        # "USRP\nTransmitter"
        n248 = Get Queue Status(queue=w593, error in (no error)=w592) -> (queue out=w600:refnum<queue>, error out=w599:errorcluster, # elements in queue=w602:i32)  [unwired: 1 in, 5 out]
        n249 = Not Equal To 0?(x=w602) -> (x != 0?=w601:bool)
        n250 = case shown="True" w601 {
          tunnel: w600 -> [_ w608]
          tunnel: w599 -> [w603 w607]
          tunnel: [w604 w606] -> w594
          tunnel: [w603 w605] -> w591
          tunnel: w590 -> [w604 _]
          frame False {
          }
          frame True {
            n251 = Dequeue Element(queue=w608, error in (no error)=w607) -> (element=w606:cluster{"t0":dbl, "dt":dbl, "Y":cdb[]}, error out=w605:errorcluster)  [unwired: 1 in, 2 out]
          }
        }
        n252 = global read "var_stop.vi" "system stop"() -> (w589:bool)
        n253 = call-poly <instrlib>:"niUSRP Write Tx Data (poly).vi"("session handle"=w595, "data"=w594, "error in (no error)"=w596) -> ("session handle out"=w597:refnum<k15>, "error out"=w598:errorcluster)  [unwired: 11 in]
      }
      n254 = call <instrlib>:"niUSRP Close Session.vi"("session handle"=w188, "error in (no error)"=w189) -> ()  [unwired: 13 in, 1 out]
      n255 = Initialize Array(cdb 0.0+0.0i, 1024 ("dimension size")) -> (w152:cdb[])
      n256 = while {
        tunnel: w190 -> [w623]
        shift-right: [w620] -> _
        shift-left: errorcluster {"status"=FALSE, "code"=0, "source"=""} ("error out") -> [w626]
        tunnel: w185 -> [w619]
        shift-right: [w618] -> _
        shift-left: errorcluster {"status"=FALSE, "code"=0, "source"=""} ("error out") -> [w617]
        tunnel: w157 -> [w615]
        tunnel: w160 -> [w614]
        tunnel: w159 -> [w613]
        tunnel: w152 -> [w612]
        shift-right: [w610] -> _
        shift-left: w147 -> [w611]
        tunnel: "Ratio of  redundant" -> [w609]
        stop <- w616 stop-if-true
        n257 = Get Queue Status(queue=w623, error in (no error)=w626) -> (queue out=w621:refnum<queue>, error out=w622:errorcluster, # elements in queue=w625:i32)  [unwired: 1 in, 5 out]
        n258 = Not Equal To 0?(x=w625) -> (x != 0?=w624:bool)
        n259 = case shown="True" w624 {
          tunnel: w622 -> [w629 w672]
          tunnel: w621 -> [_ w671]
          tunnel: [w629 w670] -> w620
          tunnel: w619 -> [_ w665]
          tunnel: [w628 w664] -> w618
          tunnel: w617 -> [w628 w663]
          tunnel: w615 -> [_ w661]
          tunnel: w614 -> [_ w660]
          tunnel: w613 -> [_ w659]
          tunnel: w612 -> [_ w649]
          tunnel: w611 -> [w627 w634]
          tunnel: [w627 w636] -> w610
          tunnel: w609 -> [_ w631]
          frame False {
          }
          frame True {
            # "length"
            # "Waveform \nGenerator"
            n260 = Dequeue Element(queue=w671, error in (no error)=w672) -> (element=w646:i16[], error out=w670:errorcluster)  [unwired: 1 in, 2 out]
            n261 = Quotient & Remainder(x=w634, y=w631) -> (x-y*floor(x/y)=w630:i32)  [unwired: 1 out]
            n262 = Unbundle(w661) -> ("samples per symbol (16)"=w655:i32, "symbol map"=w648:cdb[])  [unwired: 1 out]
            n263 = Equal?(x=w630, y=0) -> (x = y?=w632:bool)
            "x = y?" <- w632
            n264 = case shown="True" w632 {
              tunnel: [u8[] [104, 61, 1, 89, 100, 94, 186, 50] ("Array 2") u8[] [53, 187, 37, 71, 79, 49, 4, 63] ("Array 2")] -> w635
              frame False {
              }
              frame True {
              }
            }
            n265 = Increment(x=w634) -> (x+1=w636:i32)
            n266 = Array Size(array=w646) -> (size(s)=w657:i32)
            n267 = To Unsigned Word Integer(number=w657) -> (unsigned 16bit integer=w656:u16)
            n268 = Number To Boolean Array(number=w656) -> (Boolean array=w669:bool[])
            n269 = Reshape Array(w669, 2 ("dimension size"), 8 ("dimension size")) -> (w666:bool[][])
            n270 = for {
              tunnel: w666 -> [w677] mode=indexing
              tunnel: [w675] -> w658 mode=indexing
              n271 = Boolean Array To Number(Boolean array=w677) -> (number=w676:u32)
              n272 = To Unsigned Byte Integer(number=w676) -> (unsigned 8bit integer=w675:u8)
            }
            n273 = Build Array (concatenate)(w635, w658, w658, w646) -> (w662:i16[])
            n274 = call "tx_pduGen.vi"("byte array"=w662) -> ("packet bits length"=w637:i32, "pdu"=w639:i32[])  [unwired: 3 in]
            "packet bits length" <- w637
            n275 = local write "packet bits"(w639) -> ()
            n276 = local write "packet bits length"(w637) -> ()
            n277 = call "sub_bits_to_symbols.vi"("symbol map"=w648, "bits"=w639) -> ("symbols"=w647:cdb[])  [unwired: 9 in]
            n278 = Build Array (concatenate)(w647, w649) -> (w645:cdb[])
            n279 = call-poly <vilib>:"MT Pulse Shaping Filter.vi"("symbols"=w645, "pulse shaping filter coefficients"=w660, "samples per symbol (16)"=w655, "symbol rate (Hz)"=w659, "reset? (T)"=FALSE) -> ("output complex waveform"=w654:T7)  [unwired: 9 in, 1 out]
            n280 = Divide(x="Transmit power (db)", y=20.0) -> (x/y=w642:dbl)
            n281 = Unbundle(w654) -> ("t0"=w653:dbl, "dt"=w652:dbl, "Y"=w641:cdb[])
            n282 = Power Of 10(x=w642) -> (10^x=w640:dbl)
            n283 = Multiply(x=w641, y=w640) -> (x*y=w638:cdb[])
            n284 = Bundle(cluster=w654, "t0"=w653, "dt"=w652, "Y"=w638) -> (w651:T7)
            n285 = Enqueue Element(queue=w665, element=w651, error in (no error)=w663) -> (error out=w664:errorcluster)  [unwired: 1 in, 2 out]
            "Numeric 2" <- w634
          }
        }
        n286 = global read "var_stop.vi" "system stop"() -> (w616:bool)
      }
      n287 = call <instrlib>:"niUSRP Abort.vi"("session handle"=w171, "error in (no error)"=w170) -> ("session handle out"=w177:refnum<k15>, "error out"=w176:errorcluster)  [unwired: 12 in]
      n288 = call <instrlib>:"niUSRP Close Session.vi"("session handle"=w177, "error in (no error)"=w176) -> ()  [unwired: 13 in, 1 out]
    }
    frame Error {
    }
  }
  n289 = Unbundle(w6) -> ("symbol map"=w8:cdb[])  [unwired: 2 out]
  n290 = global write "var_stop.vi" "system stop"(FALSE) -> ()
  n291 = call "sub_bits_to_symbols.vi"("symbol map"=w8, "bits"=i16[] [1, 0, 1, 0, 1, 1, 0, 0, 1, 1, 0, 1, 1, 1, 0, 1, 1, 0, 1, 0, 0, 1, 0, 0, 1, 1, 1, 0, 0, 0, 1, 0, 1, 1, 1, 1, 0, 0, 1, 0, 1, 0, 0, 0, 1, 1, 0, 0, 0, 0, 1, 0, 0, 0, 0, 0, 1, 1, 1, 1, 1, 1, 0, 0] ("preamble(64) 2")) -> ("symbols"=w7:cdb[])  [unwired: 9 in]
  n292 = local write "packet bits 2"("packet bits 2") -> ()
  n293 = local write "random bits 2"("random bits 2") -> ()
  n294 = Divide(x="IQ rate 2", y="samples per symbol (16) 2") -> (x/y=w22:dbl)
  n295 = Merge Errors(w18, w17) -> (w16:errorcluster)
  n296 = Reciprocal(x=w44) -> (1/x=w43:dbl)
  n297 = Obtain Queue(element data type=i8[] [] ("output bit stream")) -> (queue out=w28:refnum<queue>)  [unwired: 4 in, 2 out]
  n298 = Obtain Queue(element data type=i16[] []) -> (queue out=w56:refnum<queue>)  [unwired: 4 in, 2 out]
  n299 = Logarithm Base 2(1:"M-PSK (4) 2") -> (0:w3:dbl)
  n300 = Obtain Queue(element data type=cluster{"t0":dbl, "dt":dbl, "Y":cdb[]} {"t0"=0.0, "dt"=0.0, "Y"=[]} ("data")) -> (queue out=w32:refnum<queue>)  [unwired: 4 in, 2 out]
  n301 = Obtain Queue(element data type=cluster{"t0":dbl, "dt":dbl, "Y":cdb[]} {"t0"=0.0, "dt"=0.0, "Y"=[]} ("data")) -> (queue out=w29:refnum<queue>)  [unwired: 4 in, 2 out]
  n302 = Obtain Queue(element data type=cluster{"t0":dbl, "dt":dbl, "Y":cdb[]} {"t0"=0.0, "dt"=1.0, "Y"=[]} ("data")) -> (queue out=w47:refnum<queue>)  [unwired: 4 in, 2 out]
  n303 = case shown="No Error" w16 {
    tunnel: w56 -> [w771 _]
    tunnel: w47 -> [w766 _]
    tunnel: w46 -> [w767 _]
    tunnel: w43 -> [w760 _]
    tunnel: w33 -> [w755 _]
    tunnel: w32 -> [w749 _]
    tunnel: w29 -> [w745 _]
    tunnel: w28 -> [w743 _]
    tunnel: w6 -> [w737 _]
    tunnel: w23 -> [w740 _]
    tunnel: w22 -> [w739 _]
    tunnel: w21 -> [w738 _]
    tunnel: w7 -> [w731 _]
    tunnel: w3 -> [w729 _]
    frame No Error {
      w727 = 0
      w728 = 0
      # "USRP interface"
      n304 = call <instrlib>:"niUSRP Initiate.vi"("session handle"=w755, "error in (no error)"=errorcluster {"status"=FALSE, "code"=0, "source"=""}) -> ("session handle out"=w754:refnum<k15>, "error out"=w753:errorcluster)  [unwired: 12 in]
      n305 = while {
        tunnel: w743 -> [w793]
        shift-right: [w786] -> _
        shift-left: errorcluster {"status"=FALSE, "code"=0, "source"=""} ("error out") -> [w792]
        shift-right: [w781] -> _
        shift-left: w728 -> [w784]
        shift-right: [w782] -> _
        shift-left: w728 -> [w783]
        tunnel: w729 -> [w778]
        shift-right: [w775] -> _
        shift-left: w728 -> [w777]
        shift-right: [w774] -> _
        shift-left: w728 -> [w776]
        stop <- w791 stop-if-true
        n306 = Get Queue Status(queue=w793, error in (no error)=w792) -> (queue out=w788:refnum<queue>, error out=w787:errorcluster, # elements in queue=w790:i32)  [unwired: 1 in, 5 out]
        n307 = local read "packet bits length 2"() -> (w779:i32)
        n308 = local read "random bits 2"() -> (w785:i8[])
        n309 = Not Equal To 0?(x=w790) -> (x != 0?=w789:bool)
        n310 = case shown="True" w789 {
          tunnel: w788 -> [_ w835]
          tunnel: w787 -> [w798 w834]
          tunnel: [w798 w829] -> w786
          tunnel: w785 -> [_ w826]
          tunnel: w784 -> [w797 w822]
          tunnel: [w797 w821] -> w781
          tunnel: [w796 w819] -> w782
          tunnel: w783 -> [w796 w820]
          tunnel: w779 -> [_ w811]
          tunnel: w778 -> [_ w807]
          tunnel: w777 -> [w795 w803]
          tunnel: [w795 w802] -> w775
          tunnel: w776 -> [w794 w801]
          tunnel: [w794 w799] -> w774
          frame False {
          }
          frame True {
            w815 = 0
            w832 = 8 ("y")
            n311 = Dequeue Element(queue=w835, error in (no error)=w834) -> (element=w812:i8[], error out=w829:errorcluster)  [unwired: 1 in, 2 out]
            n312 = Array Size(array=w812) -> (size(s)=w806:i32)
            n313 = Subtract(x=w811, y=w806) -> (x-y=w810:i32)
            n314 = Array Subset(array=w826, index=0, length=w806) -> (w813:i8[])
            n315 = Quotient & Remainder(x=w810, y=w807) -> (x-y*floor(x/y)=w816:dbl)  [unwired: 1 out]
            n316 = Not Equal?(x=w813, y=w812) -> (x != y?=w825:bool[])
            n317 = Initialize Array(0, w816) -> (w814:i32[])
            n318 = Boolean To (0,1)(Boolean=w825) -> (0, 1=w824:i16[])
            n319 = Add Array Elements(numeric array=w824) -> (sum=w823:i16)
            n320 = Quotient & Remainder(x=w806, y=w807) -> (floor(x/y)=w800:dbl)  [unwired: 1 out]
            n321 = Insert Into Array(array=w814, index=w815, new element=w813) -> (w809:i32[])
            n322 = Insert Into Array(array=w814, index=w815, new element=w812) -> (w808:i32[])
            n323 = Quotient & Remainder(x=w806, y=w832) -> (floor(x/y)=w831:i32)  [unwired: 1 out]
            n324 = Add(x=w822, y=w823) -> (x+y=w821:i32)
            n325 = Add(x=w820, y=w806) -> (x+y=w819:i32)
            n326 = Not Equal To 0?(x=w812) -> (x != 0?=w833:bool[])
            n327 = Reshape Array(w809, w800, w807) -> (w805:i32[][])
            n328 = Reshape Array(w808, w800, w807) -> (w804:i32[][])
            n329 = Add(x=w800, y=w801) -> (x+y=w799:dbl)
            n330 = Reshape Array(w833, w831, w832) -> (w830:bool[][])
            n331 = for {
              tunnel: w805 -> [w843] mode=indexing
              tunnel: w804 -> [w844] mode=indexing
              shift-right: [w839] -> w802
              shift-left: w803 -> [w838]
              n332 = Not Equal?(x=w843, y=w844) -> (x != y?=w842:bool[])
              n333 = Boolean To (0,1)(Boolean=w842) -> (0, 1=w841:i16[])
              n334 = Add Array Elements(numeric array=w841) -> (sum=w840:i16)
              n335 = Not Equal To 0?(x=w840) -> (x != 0?=w837:bool)
              n336 = Boolean To (0,1)(Boolean=w837) -> (0, 1=w836:i16)
              n337 = Add(x=w836, y=w838) -> (x+y=w839:i32)
            }
            n338 = for {
              tunnel: w830 -> [w847] mode=indexing
              tunnel: [w846] -> w828 mode=indexing
              n339 = Boolean Array To Number(Boolean array=w847) -> (number=w845:u32)
              n340 = To Unsigned Byte Integer(number=w845) -> (unsigned 8bit integer=w846:u8)
            }
            n341 = Byte Array To String(unsigned byte array=w828) -> (string=→"Rx String 2":string)
          }
        }
        "error bits 2" <- w781
        "received bits 2" <- w782
        "error symbols 2" <- w775
        "received symbols 2" <- w774
        n342 = Divide(x=w775, y=w774) -> (x/y=→"ser 2":dbl)
        n343 = Divide(x=w781, y=w782) -> (x/y=→"ber 2":dbl)
        n344 = global read "var_stop.vi" "system stop"() -> (w791:bool)
      }
      n345 = while {
        tunnel: w749 -> [w940]
        shift-right: [w933] -> _
        shift-left: errorcluster {"status"=FALSE, "code"=0, "source"=""} ("error out") -> [w939]
        shift-right: [w919] -> _
        shift-left: cluster{"t0":dbl, "dt":dbl, "Y":cdb[]} {"t0"=0.0, "dt"=0.0, "Y"=[]} ("data") -> [w934]
        tunnel: w745 -> [w932]
        shift-right: [w931] -> _
        shift-left: errorcluster {"status"=FALSE, "code"=0, "source"=""} ("error out") -> [w930]
        stop <- w929 stop-if-true
        # "Energy\ndetector"
        n346 = Get Queue Status(queue=w940, error in (no error)=w939) -> (queue out=w935:refnum<queue>, error out=w936:errorcluster, # elements in queue=w938:i32)  [unwired: 1 in, 5 out]
        n347 = Not Equal To 0?(x=w938) -> (x != 0?=w937:bool)
        n348 = case shown="True" w937 {
          tunnel: w936 -> [w962 w973]
          tunnel: w935 -> [_ w972]
          tunnel: w934 -> [w961 w967]
          tunnel: [w962 w964] -> w933
          tunnel: [w961 w963] -> w926
          frame False {
          }
          frame True {
            n349 = Unbundle(w967) -> ("Y"=w970:cdb[])  [unwired: 2 out]
            n350 = Dequeue Element(queue=w972, error in (no error)=w973) -> (element=w971:cluster{"t0":dbl, "dt":dbl, "Y":cdb[]}, error out=w964:errorcluster)  [unwired: 1 in, 2 out]
            n351 = Unbundle(w971) -> ("t0"=w966:dbl, "dt"=w965:dbl, "Y"=w969:cdb[])
            n352 = Build Array (concatenate)(w970, w969) -> (w968:cdb[])
            n353 = Bundle(cluster=w967, "t0"=w966, "dt"=w965, "Y"=w968) -> (w963:cluster{"t0":dbl, "dt":dbl, "Y":cdb[]})
          }
        }
        n354 = call "rx_ed.vi"("Wavefrom"=w926) -> ("first pulse"=w916:i32, "length"=w927:i32[], "start index"=w928:i32[])  [unwired: 8 in]
        n355 = for {
          tunnel: w932 -> [w948]
          tunnel: w926 -> [w945]
          shift-right: [w947] -> w931
          shift-left: w930 -> [w946]
          tunnel: w928 -> [w944] mode=indexing
          tunnel: w927 -> [w943] mode=indexing
          tunnel: [w944] -> w922
          tunnel: [w943] -> w921
          n356 = Greater Or Equal?(x=w943, y=128) -> (x >= y?=w941:bool)
          n357 = case shown="True" w941 {
            tunnel: w948 -> [_ w960]
            tunnel: [w949 w959] -> w947
            tunnel: w946 -> [w949 w958]
            tunnel: w945 -> [_ w957]
            tunnel: w944 -> [_ w951]
            tunnel: w943 -> [_ w950]
            frame False {
            }
            frame True {
              n358 = Unbundle(w957) -> ("t0"=w955:dbl, "dt"=w956:dbl, "Y"=w953:cdb[])
              n359 = Array Subset(array=w953, index=w951, length=w950) -> (w952:cdb[])
              n360 = Bundle("t0"=w955, "dt"=w956, w952) -> (w954:cluster{"t0":dbl, "dt":dbl, cdb[]})  [unwired: 1 in]
              n361 = Enqueue Element(queue=w960, element=w954, error in (no error)=w958) -> (error out=w959:errorcluster)  [unwired: 1 in, 2 out]
            }
          }
        }
        n362 = Add(x=w922, y=w921) -> (x+y=w918:i32)
        n363 = Max & Min(x=w918, y=w916) -> (max(x,y)=w917:i32)  [unwired: 1 out]
        n364 = Unbundle(w926) -> ("t0"=w925:dbl, "dt"=w924:dbl, "Y"=w923:cdb[])
        n365 = global read "var_stop.vi" "system stop"() -> (w929:bool)
        n366 = Array Subset(array=w923, index=w917) -> (w920:cdb[])  [unwired: 1 in]
        n367 = Bundle(cluster=w926, "t0"=w925, "dt"=w924, "Y"=w920) -> (w919:cluster{"t0":dbl, "dt":dbl, "Y":cdb[]})
      }
      n368 = while {
        tunnel: w745 -> [w861]
        shift-right: [w855] -> _
        shift-left: errorcluster {"status"=FALSE, "code"=0, "source"=""} ("error out") -> [w860]
        tunnel: w743 -> [w854]
        shift-right: [w853] -> _
        shift-left: errorcluster {"status"=FALSE, "code"=0, "source"=""} ("error out") -> [w852]
        tunnel: w738 -> [w850]
        tunnel: w737 -> [w849]
        tunnel: w731 -> [w848]
        stop <- w851 stop-if-true
        # "Signal \nDemodulator"
        n369 = Get Queue Status(queue=w861, error in (no error)=w860) -> (queue out=w857:refnum<queue>, error out=w856:errorcluster, # elements in queue=w859:i32)  [unwired: 1 in, 5 out]
        n370 = Not Equal To 0?(x=w859) -> (x != 0?=w858:bool)
        n371 = case shown="True" w858 {
          tunnel: w857 -> [_ w894]
          tunnel: w856 -> [w863 w895]
          tunnel: [w863 w893] -> w855
          tunnel: w854 -> [_ w886]
          tunnel: [w862 w885] -> w853
          tunnel: w852 -> [w862 w884]
          tunnel: w850 -> [_ w873]
          tunnel: w849 -> [_ w877]
          tunnel: w848 -> [_ w869]
          frame False {
          }
          frame True {
            # "cross+eq"
            n372 = Unbundle(w877) -> ("samples per symbol (16) 2"=w876:i32, "symbol map"=w875:cdb[], "index map"=w874:u32[])
            n373 = Dequeue Element(queue=w894, error in (no error)=w895) -> (element=w868:cluster{"t0":dbl, "dt":dbl, "Y":cdb[]}, error out=w893:errorcluster)  [unwired: 1 in, 2 out]
            n374 = Unbundle(w868) -> ("Y"=w867:cdb[])  [unwired: 2 out]
            n375 = Bundle By Name("Y"=w867) -> (w872:waveform(cdb))  [unwired: 1 in]
            n376 = call-poly <vilib>:"FFT Power Spectrum and PSD.vi"("dB On (F)"=TRUE, "time signal"=w872) -> ("Power Spectrum / PSD"=→"Spectrum monitor 2":cluster{"f0":dbl, "df":dbl, "magnitude":dbl[]})  [unwired: 6 in, 3 out]
            n377 = call-poly <vilib>:"MT Matched Filter.vi"("input complex waveform"=w868, "matched filter coefficients"=w873, "samples per symbol (16)"=w876, "reset? (T)"=FALSE) -> ("output complex waveform"=w892:T7, "error out"=w891:errorcluster)  [unwired: 10 in]
            n378 = call-poly <vilib>:"MT Align To Ideal Symbols.vi"("input complex waveform"=w892, "matched filter coefficients"=w873, "samples per symbol (16)"=w876, "error in (no error)"=w891, "reset? (T)"=FALSE) -> ("output complex waveform"=w889:T7, "error out"=w890:errorcluster)  [unwired: 8 in, 1 out]
            n379 = call <vilib>:"MT Decimate Oversampled Waveform.vi"("input complex waveform"=w889, "decimation factor"=w876, "error in (no error)"=w890, "reset? (T)"=FALSE) -> ("output complex waveform"=w888:T7)  [unwired: 10 in, 1 out]
            n380 = Unbundle(w888) -> ("Y"=w866:cdb[])  [unwired: 2 out]
            n381 = call "rx_ceEq.vi"("preamble"=w869, "symbols"=w866) -> ("valid?"=w882:bool, "eq symbols"=w883:cdb[])
            "valid? 2" <- w882
            n382 = case shown="True" w882 {
              tunnel: [i8[] [] ("output bit stream") w900] -> w865
              tunnel: w875 -> [_ w901]
              tunnel: w883 -> [_ w898]
              tunnel: w874 -> [_ w899]
              tunnel: w866 -> [_ w897]
              frame False {
              }
              frame True {
                n383 = local read "Modulation 2"() -> (w902:enum16{"PSK", "QAM"})
                n384 = case shown="\"PSK\", Default" w902 {
                  tunnel: w898 -> [w906 w909]
                  tunnel: w901 -> [w905 w908]
                  tunnel: [w903 w907] -> w900
                  tunnel: w899 -> [w904 _]
                  frame "PSK", Default {
                    n385 = call "sub_psk_demod.vi"("index map"=w904, "symbol map"=w905, "symbol"=w906) -> ("bitstream"=w903:i16[])  [unwired: 8 in]
                  }
                  frame "QAM" {
                    n386 = call "sub_qam_demod.vi"("symbol map"=w908, "symbol"=w909) -> ("bitstream"=w907:i16[])  [unwired: 9 in]
                  }
                }
                "RX Constellation Map 2" <- w898
                "RX Constellation Map (uneq) 2" <- w897
              }
            }
            n387 = call "rx_pduExtract.vi"("output bit stream"=w865) -> ("found?"=w887:bool, "packet len"=w881:u32, "ppdu"=w864:i8[])  [unwired: 2 in]
            "found? 2" <- w887
            n388 = case shown="True" w887 {
              tunnel: w864 -> [_ w913]
              tunnel: w886 -> [_ w915]
              tunnel: [w910 w914] -> w885
              tunnel: w884 -> [w910 w911]
              tunnel: w881 -> [_ w912]
              frame False {
              }
              frame True {
                n389 = Enqueue Element(queue=w915, element=w913, error in (no error)=w911) -> (error out=w914:errorcluster)  [unwired: 1 in, 2 out]
                "packet len 2" <- w912
              }
            }
          }
        }
        n390 = global read "var_stop.vi" "system stop"() -> (w851:bool)
      }
      n391 = Initialize Array(cdb 0.0+0.0i, 25000 ("dimension size")) -> (w761:cdb[])
      n392 = while {
        tunnel: w771 -> [w1096]
        shift-right: [w1094] -> _
        shift-left: errorcluster {"status"=FALSE, "code"=0, "source"=""} ("error out") -> [w1095]
        shift-right: [w1092] -> _
        shift-left: -1111 -> [w1093]
        shift-right: [w1089] -> _
        shift-left: w727 -> [w1090]
        tunnel: "Ratio of  redundant 2" -> [w1088]
        stop <- "stop 2" stop-if-true
        n393 = Wait Until Next ms Multiple(millisecond multiple="millisecond multiple 2") -> ()  [unwired: 1 out]
        n394 = global write "var_stop.vi" "system stop"("stop 2") -> ()
        n395 = case shown="True" "Keep sending 2" {
          tunnel: w1096 -> [_ w1121]
          tunnel: w1095 -> [w1100 w1120]
          tunnel: [w1100 w1119] -> w1094
          tunnel: w1093 -> [w1099 w1116]
          tunnel: [w1099 w1115] -> w1092
          tunnel: w1090 -> [w1098 w1101]
          tunnel: [w1098 w1106] -> w1089
          tunnel: w1088 -> [_ w1107]
          frame False {
          }
          frame True {
            w1113 = 8
            n396 = call-poly <vilib>:"MT Generate Bits (poly).vi"("total bits (128)"="random bits length 2", "seed in (0xD6BF7DF2)"=w1116, "reset? (T)"=FALSE) -> ("output bit stream"=w1103:i8[], "seed out"=w1115:i32)  [unwired: 10 in, 1 out]
            n397 = Not Equal To 0?(x=w1103) -> (x != 0?=w1108:bool[])
            n398 = Array Size(array=w1108) -> (size(s)=w1112:i32)
            n399 = Divide(x=w1112, y=w1113) -> (x/y=w1111:dbl)
            n400 = Reshape Array(w1108, w1111, w1113) -> (w1110:bool[][])
            n401 = for {
              tunnel: w1110 -> [w1126] mode=indexing
              tunnel: [w1124] -> w1109 mode=indexing
              n402 = Boolean Array To Number(Boolean array=w1126) -> (number=w1125:u32)
              n403 = To Unsigned Byte Integer(number=w1125) -> (unsigned 8bit integer=w1124:u8)
            }
            n404 = Increment(x=w1101) -> (x+1=w1106:i32)
            n405 = Array Size(array=w1109) -> (size(s)=w1118:i32)
            n406 = Quotient & Remainder(x=w1101, y=w1107) -> (x-y*floor(x/y)=w1102:i32)  [unwired: 1 out]
            n407 = Not Equal To 0?(x=w1118) -> (x != 0?=w1122:bool)
            n408 = Equal?(x=w1102, y=0) -> (x = y?=w1104:bool)
            n409 = case shown="True" w1122 {
              tunnel: w1109 -> [_ w1128]
              tunnel: w1121 -> [_ w1131]
              tunnel: w1120 -> [w1127 w1130]
              tunnel: [w1127 w1129] -> w1119
              frame False {
              }
              frame True {
                n410 = Enqueue Element(queue=w1131, element=w1128, error in (no error)=w1130) -> (error out=w1129:errorcluster)  [unwired: 1 in, 2 out]
              }
            }
            n411 = case shown="True" w1104 {
              tunnel: w1103 -> [_ w1123]
              frame False {
              }
              frame True {
                n412 = local write "random bits 2"(w1123) -> ()
              }
            }
            "Numeric 4" <- w1101
          }
        }
      }
      n413 = while {
        tunnel: w754 -> [w992]
        shift-right: [w980] -> w750
        shift-left: w753 -> [w991]
        tunnel: w749 -> [w989]
        shift-right: [w983] -> _
        shift-left: errorcluster {"status"=FALSE, "code"=0, "source"=""} ("error out") -> [w988]
        tunnel: [w981] -> w751
        i -> [w978]
        stop <- w979 stop-if-true
        # "USRP\nReceiver"
        n414 = Get Queue Status(queue=w989, error in (no error)=w988) -> (queue out=w985:refnum<queue>, error out=w984:errorcluster, # elements in queue=w987:i32)  [unwired: 1 in, 5 out]
        "# elements in queue 2" <- w987
        n415 = Less?(x=w987, y=5000) -> (x < y?=w976:bool)
        n416 = Greater Or Equal?(x=w978, y=25) -> (x >= y?=w975:bool)
        n417 = And(x=w976, y=w975) -> (x .and. y?=w974:bool)
        n418 = call-poly <instrlib>:"niUSRP Fetch Rx Data (poly).vi"("session handle"=w992, "number of samples"="number of samples 2", "error in (no error)"=w991) -> ("session handle out"=w981:refnum<k15>, "data"=w982:cluster{"t0":dbl, "dt":dbl, "Y":cdb[]}, "error out"=w980:errorcluster)  [unwired: 9 in, 1 out]
        n419 = case shown="False" w974 {
          tunnel: w985 -> [_ w997]
          tunnel: w984 -> [w993 w996]
          tunnel: [w993 w995] -> w983
          tunnel: w982 -> [_ w994]
          frame False {
          }
          frame True {
            n420 = Enqueue Element(queue=w997, element=w994, error in (no error)=w996) -> (error out=w995:errorcluster)  [unwired: 1 in, 2 out]
          }
        }
        n421 = global read "var_stop.vi" "system stop"() -> (w979:bool)
      }
      n422 = Bundle(0.0, w760, w761) -> (w758:cluster{dbl, dbl, cdb[]})  [unwired: 1 in]
      n423 = while {
        shift-right: [w1007] -> w770
        shift-left: errorcluster {"status"=FALSE, "code"=0, "source"=""} ("error out") -> [w1005]
        tunnel: [w1006] -> w769
        tunnel: w767 -> [w1004]
        tunnel: w766 -> [w1002]
        shift-right: [w1000] -> _
        shift-left: errorcluster {"status"=FALSE, "code"=0, "source"=""} ("error out") -> [w1001]
        tunnel: w758 -> [w999]
        stop <- w998 stop-if-true
        # "USRP\nTransmitter"
        n424 = Get Queue Status(queue=w1002, error in (no error)=w1001) -> (queue out=w1009:refnum<queue>, error out=w1008:errorcluster, # elements in queue=w1011:i32)  [unwired: 1 in, 5 out]
        n425 = Not Equal To 0?(x=w1011) -> (x != 0?=w1010:bool)
        n426 = case shown="True" w1010 {
          tunnel: w1009 -> [_ w1017]
          tunnel: w1008 -> [w1012 w1016]
          tunnel: [w1013 w1015] -> w1003
          tunnel: [w1012 w1014] -> w1000
          tunnel: w999 -> [w1013 _]
          frame False {
          }
          frame True {
            n427 = Dequeue Element(queue=w1017, error in (no error)=w1016) -> (element=w1015:cluster{"t0":dbl, "dt":dbl, "Y":cdb[]}, error out=w1014:errorcluster)  [unwired: 1 in, 2 out]
          }
        }
        n428 = global read "var_stop.vi" "system stop"() -> (w998:bool)
        n429 = call-poly <instrlib>:"niUSRP Write Tx Data (poly).vi"("session handle"=w1004, "data"=w1003, "error in (no error)"=w1005) -> ("session handle out"=w1006:refnum<k15>, "error out"=w1007:errorcluster)  [unwired: 11 in]
      }
      n430 = call <instrlib>:"niUSRP Abort.vi"("session handle"=w751, "error in (no error)"=w750) -> ("session handle out"=w757:refnum<k15>, "error out"=w756:errorcluster)  [unwired: 12 in]
      n431 = call <instrlib>:"niUSRP Close Session.vi"("session handle"=w757, "error in (no error)"=w756) -> ()  [unwired: 13 in, 1 out]
      n432 = call <instrlib>:"niUSRP Close Session.vi"("session handle"=w769, "error in (no error)"=w770) -> ()  [unwired: 13 in, 1 out]
      n433 = Initialize Array(cdb 0.0+0.0i, 1024 ("dimension size")) -> (w732:cdb[])
      n434 = while {
        tunnel: w771 -> [w1032]
        shift-right: [w1029] -> _
        shift-left: errorcluster {"status"=FALSE, "code"=0, "source"=""} ("error out") -> [w1035]
        tunnel: w766 -> [w1028]
        shift-right: [w1027] -> _
        shift-left: errorcluster {"status"=FALSE, "code"=0, "source"=""} ("error out") -> [w1026]
        tunnel: w737 -> [w1024]
        tunnel: w740 -> [w1023]
        tunnel: w739 -> [w1022]
        tunnel: w732 -> [w1021]
        shift-right: [w1019] -> _
        shift-left: w727 -> [w1020]
        tunnel: "Ratio of  redundant 2" -> [w1018]
        stop <- w1025 stop-if-true
        n435 = Get Queue Status(queue=w1032, error in (no error)=w1035) -> (queue out=w1030:refnum<queue>, error out=w1031:errorcluster, # elements in queue=w1034:i32)  [unwired: 1 in, 5 out]
        n436 = Not Equal To 0?(x=w1034) -> (x != 0?=w1033:bool)
        n437 = case shown="True" w1033 {
          tunnel: w1031 -> [w1038 w1081]
          tunnel: w1030 -> [_ w1080]
          tunnel: [w1038 w1079] -> w1029
          tunnel: w1028 -> [_ w1074]
          tunnel: [w1037 w1073] -> w1027
          tunnel: w1026 -> [w1037 w1072]
          tunnel: w1024 -> [_ w1070]
          tunnel: w1023 -> [_ w1069]
          tunnel: w1022 -> [_ w1068]
          tunnel: w1021 -> [_ w1058]
          tunnel: w1020 -> [w1036 w1043]
          tunnel: [w1036 w1045] -> w1019
          tunnel: w1018 -> [_ w1040]
          frame False {
          }
          frame True {
            # "length"
            # "Waveform \nGenerator"
            n438 = Dequeue Element(queue=w1080, error in (no error)=w1081) -> (element=w1055:i16[], error out=w1079:errorcluster)  [unwired: 1 in, 2 out]
            n439 = Quotient & Remainder(x=w1043, y=w1040) -> (x-y*floor(x/y)=w1039:i32)  [unwired: 1 out]
            n440 = Unbundle(w1070) -> ("samples per symbol (16) 2"=w1064:i32, "symbol map"=w1057:cdb[])  [unwired: 1 out]
            n441 = Equal?(x=w1039, y=0) -> (x = y?=w1041:bool)
            "x = y? 2" <- w1041
            n442 = case shown="True" w1041 {
              tunnel: [u8[] [104, 61, 1, 89, 100, 94, 186, 50] ("Array 2") u8[] [53, 187, 37, 71, 79, 49, 4, 63] ("Array 2")] -> w1044
              frame False {
              }
              frame True {
              }
            }
            n443 = Increment(x=w1043) -> (x+1=w1045:i32)
            n444 = Array Size(array=w1055) -> (size(s)=w1066:i32)
            n445 = To Unsigned Word Integer(number=w1066) -> (unsigned 16bit integer=w1065:u16)
            n446 = Number To Boolean Array(number=w1065) -> (Boolean array=w1078:bool[])
            n447 = Reshape Array(w1078, 2 ("dimension size"), 8 ("dimension size")) -> (w1075:bool[][])
            n448 = for {
              tunnel: w1075 -> [w1086] mode=indexing
              tunnel: [w1084] -> w1067 mode=indexing
              n449 = Boolean Array To Number(Boolean array=w1086) -> (number=w1085:u32)
              n450 = To Unsigned Byte Integer(number=w1085) -> (unsigned 8bit integer=w1084:u8)
            }
            n451 = Build Array (concatenate)(w1044, w1067, w1067, w1055) -> (w1071:i16[])
            n452 = call "tx_pduGen.vi"("byte array"=w1071) -> ("packet bits length"=w1046:i32, "pdu"=w1048:i32[])  [unwired: 3 in]
            "packet bits length 2" <- w1046
            n453 = local write "packet bits 2"(w1048) -> ()
            n454 = local write "packet bits length 2"(w1046) -> ()
            n455 = call "sub_bits_to_symbols.vi"("symbol map"=w1057, "bits"=w1048) -> ("symbols"=w1056:cdb[])  [unwired: 9 in]
            n456 = Build Array (concatenate)(w1056, w1058) -> (w1054:cdb[])
            n457 = call-poly <vilib>:"MT Pulse Shaping Filter.vi"("symbols"=w1054, "pulse shaping filter coefficients"=w1069, "samples per symbol (16)"=w1064, "symbol rate (Hz)"=w1068, "reset? (T)"=FALSE) -> ("output complex waveform"=w1063:T7)  [unwired: 9 in, 1 out]
            n458 = Divide(x="Transmit power (db) 2", y=20.0) -> (x/y=w1051:dbl)
            n459 = Unbundle(w1063) -> ("t0"=w1062:dbl, "dt"=w1061:dbl, "Y"=w1050:cdb[])
            n460 = Power Of 10(x=w1051) -> (10^x=w1049:dbl)
            n461 = Multiply(x=w1050, y=w1049) -> (x*y=w1047:cdb[])
            n462 = Bundle(cluster=w1063, "t0"=w1062, "dt"=w1061, "Y"=w1047) -> (w1060:T7)
            n463 = Enqueue Element(queue=w1074, element=w1060, error in (no error)=w1072) -> (error out=w1073:errorcluster)  [unwired: 1 in, 2 out]
            "Numeric 3" <- w1043
          }
        }
        n464 = global read "var_stop.vi" "system stop"() -> (w1025:bool)
      }
    }
    frame Error {
    }
  }
